vi "Main.vi"() -> ()   [LabVIEW 2013]
uses:
  <vilib>/Utility/error.llb/DialogType.ctl
panel:
  in  "Boolean":bool
  in  "Set Output ON All":bool
  in  "Set Output OFF All":bool
  out "CURRENTSET":dbl[](array[numeric])
  in  "CurrentModulationOn":bool
  in  "Amp":dbl
  in  "CurrentModulationB":bool
  in  "ModulationUpDown":bool
  in  "ModulationNumberOfSteps":i32
  in  "ModulationState":i32
  in  "Step":dbl
  in  "Period":u32
  in  "ConnectAll":bool
  in  "DisconnectAll":bool
  in  "SetCurrentAll":bool
  in  "SetVoltageAll":bool
  in  "SetOutputOffB":bool
  in  "SetOutputOnB":bool
  in  "ReadFromFile":bool
  in  "Name":string="55"
  out "NAME":string[](array[string])
  in  "WriteToFile":bool
  in  "SetCurrent":dbl step=0.1
  in  "SetVoltage":dbl
  in  "SetCurrentB":bool
  in  "SetVoltageB":bool
  in  "DeleteChannel":bool
  in  "ConnectChannel":bool
  in  "DisconnectChannel":bool
  out "ADRESS":string[](array[string])
  out "VIRef":refnum<vi>[](array[refnum])
  in  "Quit":bool
  in  "List of channels":i32(listbox)
  in  "IP":string="172.16.21.19"
  in  "AddChannel":bool
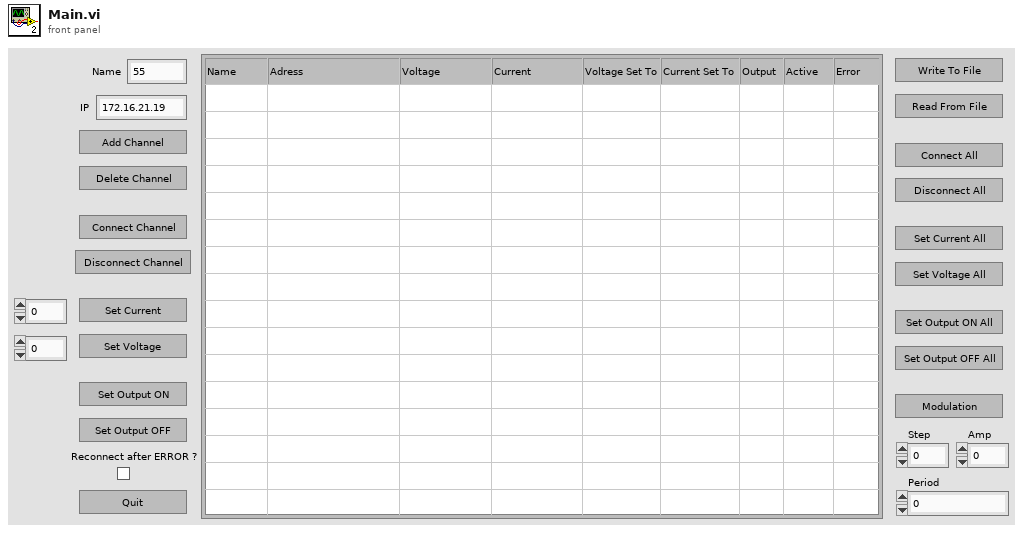
[diagram p1: front panel]
types:
  T1 = typedef "DialogType.ctl" = u16
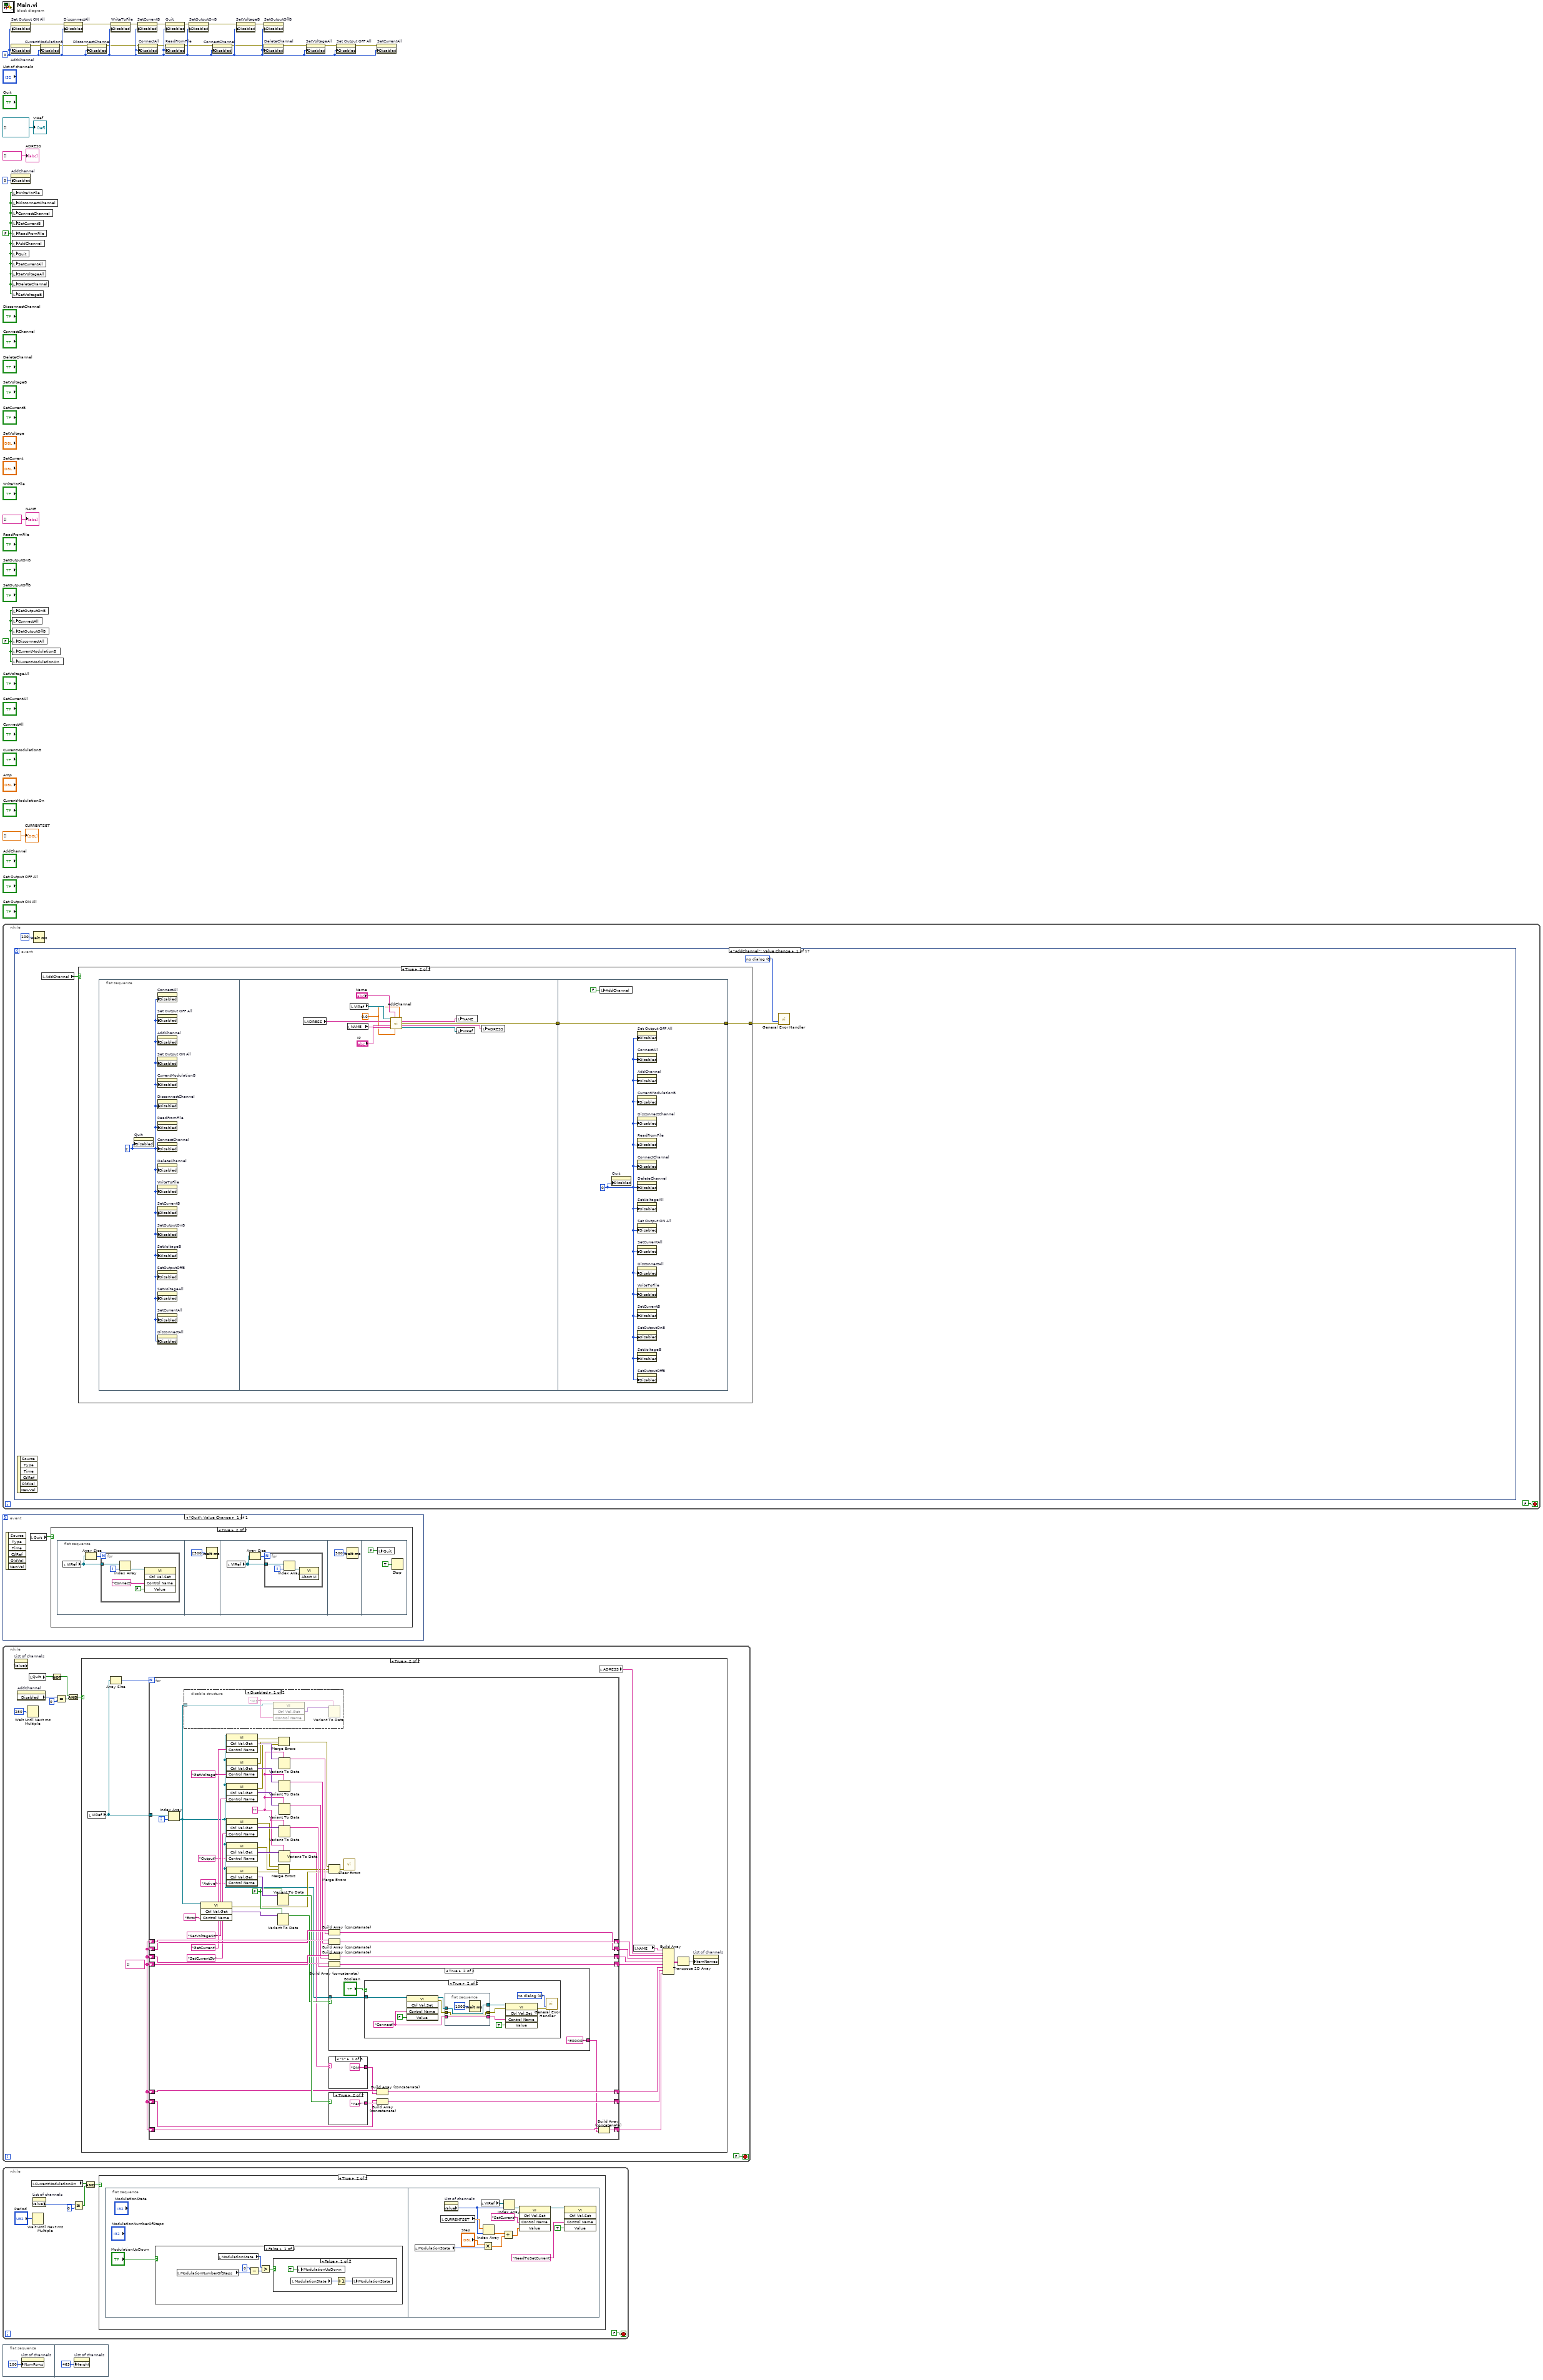
[diagram p0: block diagram]
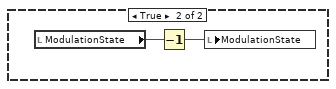
[diagram p3: hidden frame]
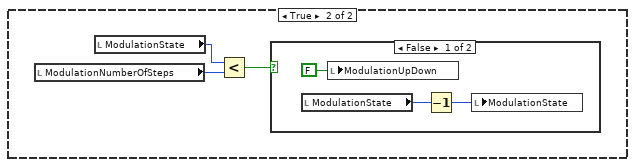
[diagram p4: hidden frame]
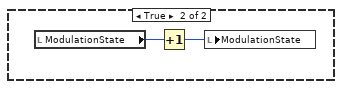
[diagram p5: hidden frame]
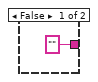
[diagram p8: hidden frame]
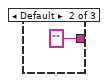
[diagram p10: hidden frame]
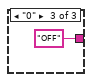
[diagram p11: hidden frame]
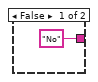
[diagram p12: hidden frame]
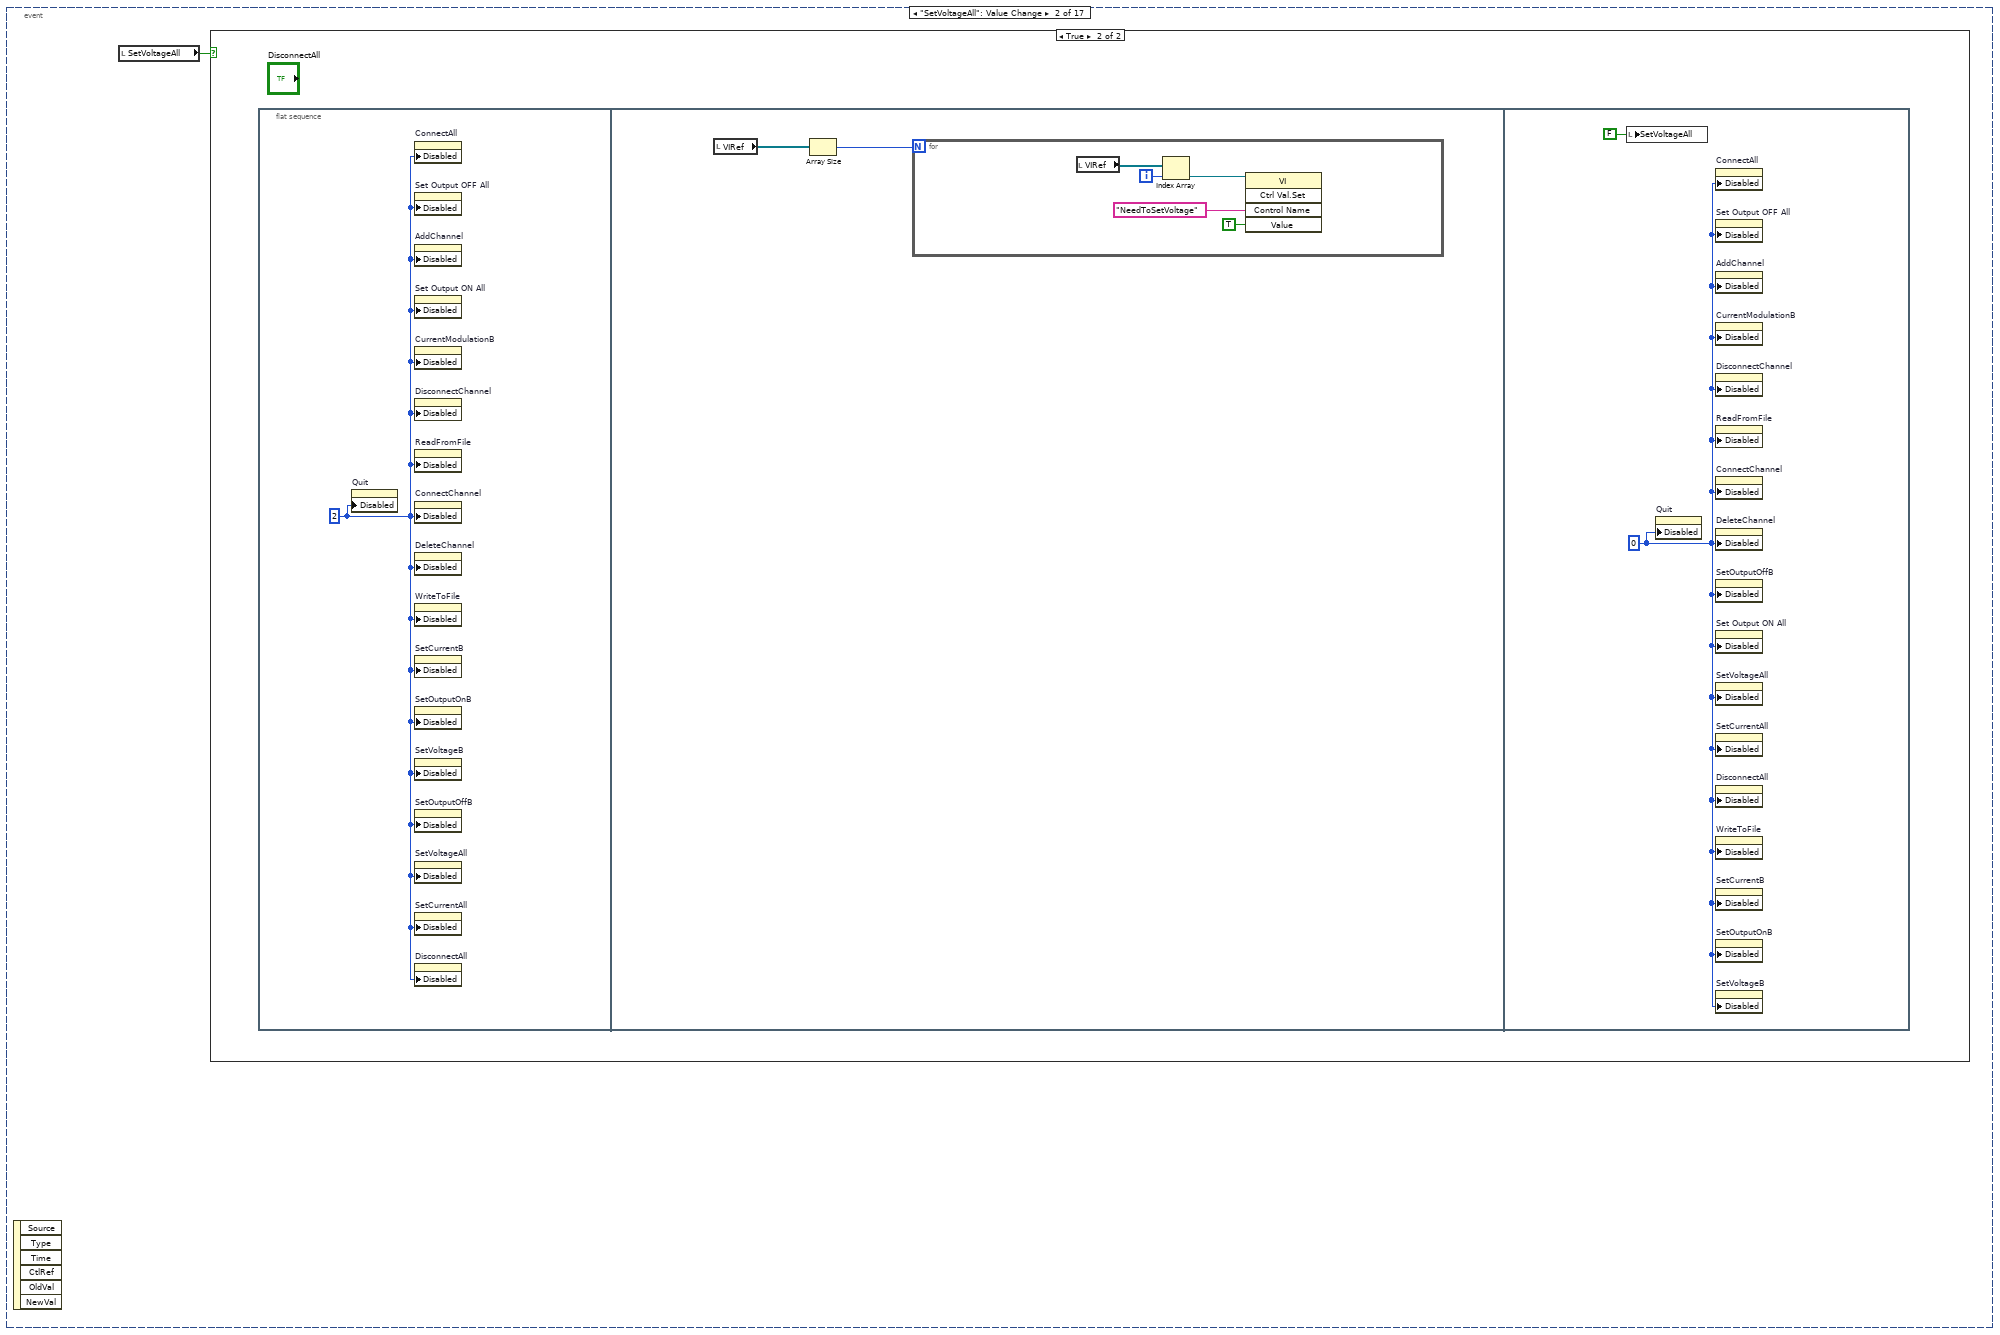
[diagram p15: hidden frame]
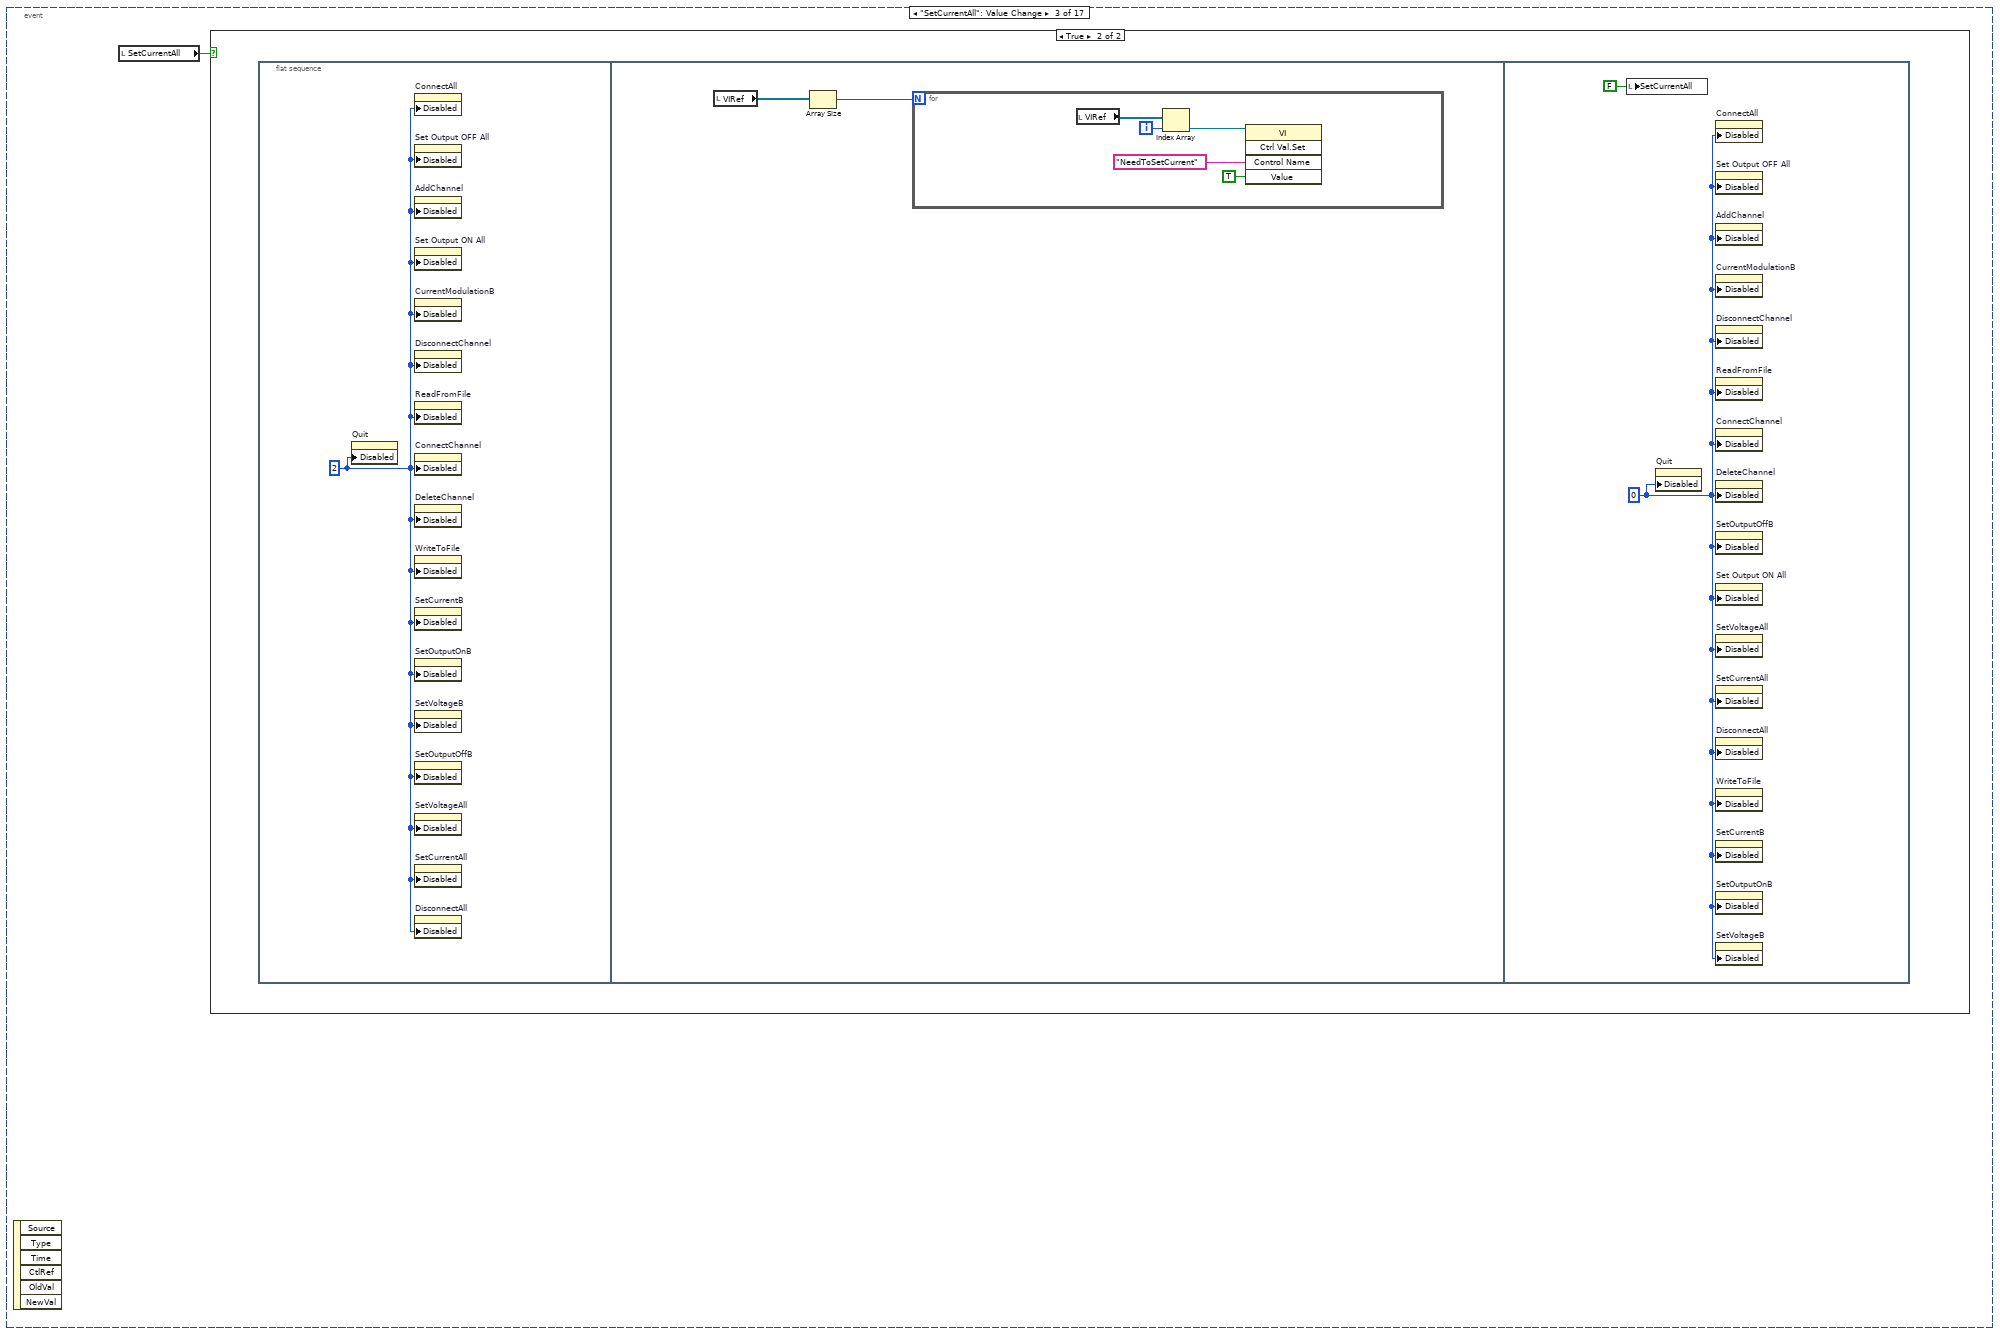
[diagram p17: hidden frame]
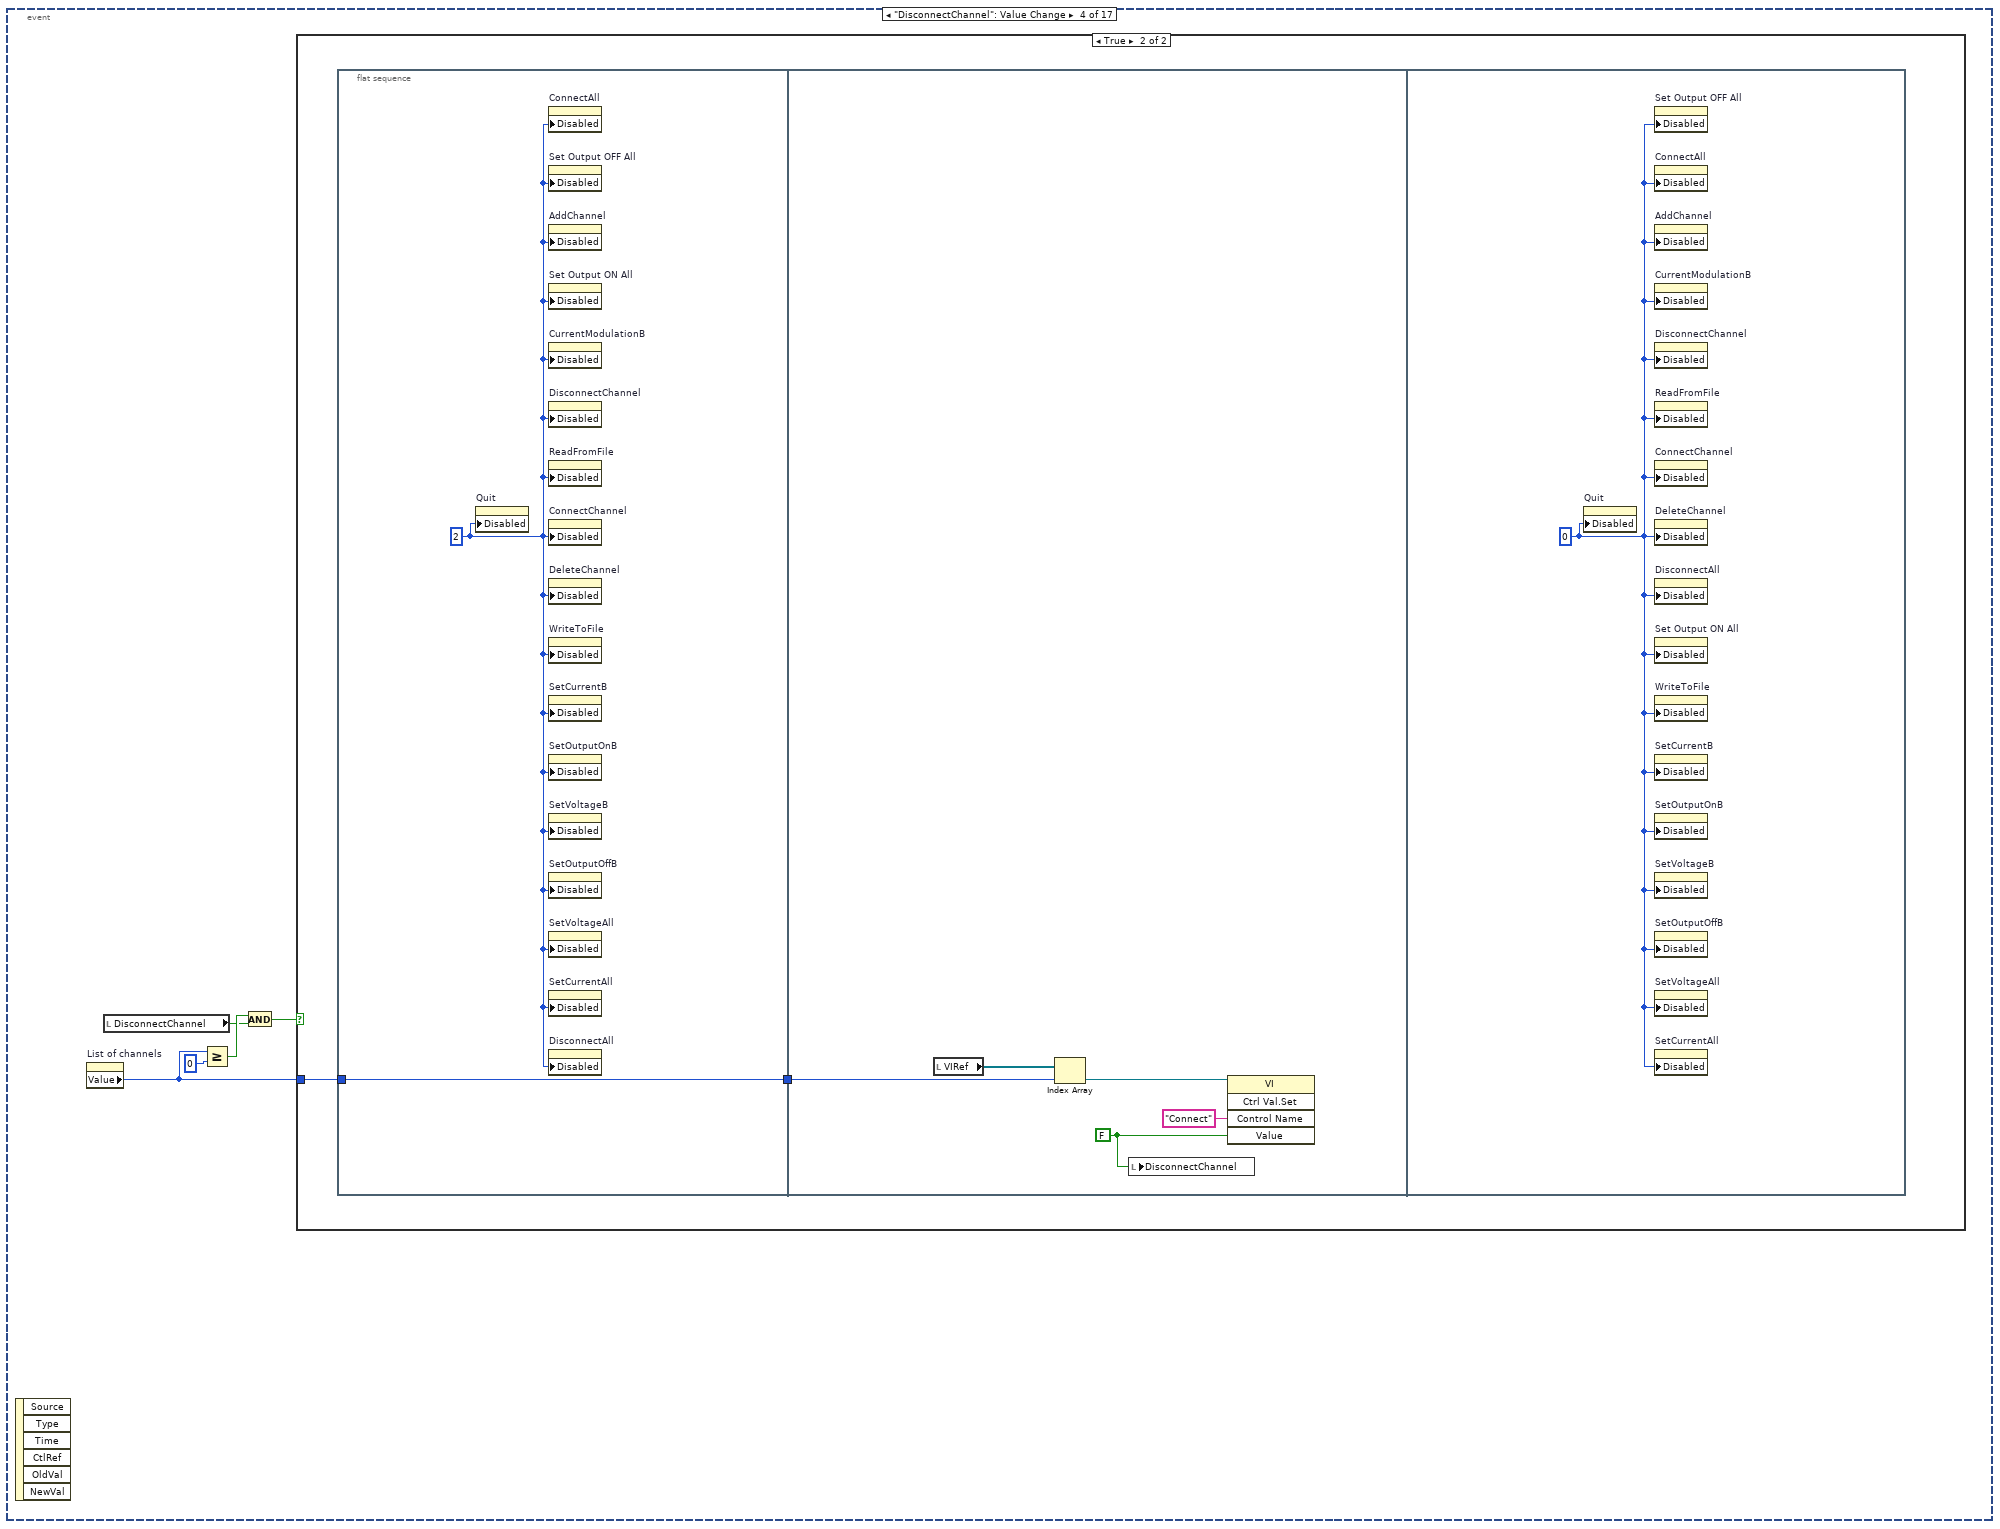
[diagram p19: hidden frame]
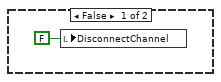
[diagram p20: hidden frame]
diagram:
  w17 = u8 0 ("Disabled")
  w19 = FALSE ("SetOutputOnB")
  w20 = FALSE ("OK Button")
  n1 = while {
    stop <- FALSE stop-if-true
    n2 = event shown="[0] \"AddChannel\": Value Change" {
      selector: _ -> [_ _ _ _ _ _ _ _ _ _ _ _ _ _ _ _ _]
      dyn-events: _ -> [_ _ _ _ _ _ _ _ _ _ _ _ _ _ _ _ _]
      timeout: _ -> [_ _ _ _ _ _ _ _ _ _ _ _ _ _ _ _ _]
      event "AddChannel": Value Change {
        w27 = T1 0 items=["no dialog", "OK message", "continue or stop message", "OK message + warnings", "continue/stop + warnings"] ("type of dialog (OK msg:1)")
        n3 = event-data() -> ()  [unwired: 7 out]
        n4 = local read "AddChannel"() -> (w29:bool)
        n5 = case shown="True" w29 {
          tunnel: [_ w30] -> w28
          frame False {
          }
          frame True {
            n6 = flat-sequence {
              tunnel: [w33] -> w31
              tunnel: [w43] -> w30
              tunnel: w31 -> [w43]
              frame #0 {
                w32 = u8 2 ("Disabled")
                n7 = property on="Quit" class="Bool (strict)"("Disabled"=w32) -> ()  [unwired: 2 in, 2 out]
                n8 = property on="ConnectAll" class="Bool (strict)"("Disabled"=w32) -> ()  [unwired: 2 in, 2 out]
                n9 = property on="Set Output OFF All" class="Bool (strict)"("Disabled"=w32) -> ()  [unwired: 2 in, 2 out]
                n10 = property on="AddChannel" class="Bool (strict)"("Disabled"=w32) -> ()  [unwired: 2 in, 2 out]
                n11 = property on="Set Output ON All" class="Bool (strict)"("Disabled"=w32) -> ()  [unwired: 2 in, 2 out]
                n12 = property on="CurrentModulationB" class="Bool (strict)"("Disabled"=w32) -> ()  [unwired: 2 in, 2 out]
                n13 = property on="DisconnectChannel" class="Bool (strict)"("Disabled"=w32) -> ()  [unwired: 2 in, 2 out]
                n14 = property on="ReadFromFile" class="Bool (strict)"("Disabled"=w32) -> ()  [unwired: 2 in, 2 out]
                n15 = property on="ConnectChannel" class="Bool (strict)"("Disabled"=w32) -> ()  [unwired: 2 in, 2 out]
                n16 = property on="DeleteChannel" class="Bool (strict)"("Disabled"=w32) -> ()  [unwired: 2 in, 2 out]
                n17 = property on="WriteToFile" class="Bool (strict)"("Disabled"=w32) -> ()  [unwired: 2 in, 2 out]
                n18 = property on="SetCurrentB" class="Bool (strict)"("Disabled"=w32) -> ()  [unwired: 2 in, 2 out]
                n19 = property on="SetOutputOnB" class="Bool (strict)"("Disabled"=w32) -> ()  [unwired: 2 in, 2 out]
                n20 = property on="SetVoltageB" class="Bool (strict)"("Disabled"=w32) -> ()  [unwired: 2 in, 2 out]
                n21 = property on="SetOutputOffB" class="Bool (strict)"("Disabled"=w32) -> ()  [unwired: 2 in, 2 out]
                n22 = property on="SetVoltageAll" class="Bool (strict)"("Disabled"=w32) -> ()  [unwired: 2 in, 2 out]
                n23 = property on="SetCurrentAll" class="Bool (strict)"("Disabled"=w32) -> ()  [unwired: 2 in, 2 out]
                n24 = property on="DisconnectAll" class="Bool (strict)"("Disabled"=w32) -> ()  [unwired: 2 in, 2 out]
              }
              frame #1 {
                w34 = 0.0 ("SetVoltage")
                n25 = local read "ADRESS"() -> (w40:string[])
                n26 = local read "NAME"() -> (w39:string[])
                n27 = local read "VIRef"() -> (w38:refnum<vi>[])
                n28 = call "AddChannel.vi"("VIRef"=w38, "Name"="Name", "SetCurrent"=w34, "ADRESS"=w40, "NAME"=w39, "Address"="IP", "SetVoltage"=w34) -> ("NAMEOut"=w35:string[], "error out"=w33:errorcluster, "ADRESSOut"=w36:string[], "VIRefOut"=w37:refnum<vi>[])  [unwired: 1 in, 4 out]
                n29 = local write "NAME"(w35) -> ()
                n30 = local write "VIRef"(w37) -> ()
                n31 = local write "ADRESS"(w36) -> ()
              }
              frame #2 {
                w44 = u8 0 ("Disabled")
                n32 = local write "AddChannel"(FALSE ("AddChannel")) -> ()
                n33 = property on="Quit" class="Bool (strict)"("Disabled"=w44) -> ()  [unwired: 2 in, 2 out]
                n34 = property on="Set Output OFF All" class="Bool (strict)"("Disabled"=w44) -> ()  [unwired: 2 in, 2 out]
                n35 = property on="ConnectAll" class="Bool (strict)"("Disabled"=w44) -> ()  [unwired: 2 in, 2 out]
                n36 = property on="AddChannel" class="Bool (strict)"("Disabled"=w44) -> ()  [unwired: 2 in, 2 out]
                n37 = property on="CurrentModulationB" class="Bool (strict)"("Disabled"=w44) -> ()  [unwired: 2 in, 2 out]
                n38 = property on="DisconnectChannel" class="Bool (strict)"("Disabled"=w44) -> ()  [unwired: 2 in, 2 out]
                n39 = property on="ReadFromFile" class="Bool (strict)"("Disabled"=w44) -> ()  [unwired: 2 in, 2 out]
                n40 = property on="ConnectChannel" class="Bool (strict)"("Disabled"=w44) -> ()  [unwired: 2 in, 2 out]
                n41 = property on="DeleteChannel" class="Bool (strict)"("Disabled"=w44) -> ()  [unwired: 2 in, 2 out]
                n42 = property on="SetVoltageAll" class="Bool (strict)"("Disabled"=w44) -> ()  [unwired: 2 in, 2 out]
                n43 = property on="Set Output ON All" class="Bool (strict)"("Disabled"=w44) -> ()  [unwired: 2 in, 2 out]
                n44 = property on="SetCurrentAll" class="Bool (strict)"("Disabled"=w44) -> ()  [unwired: 2 in, 2 out]
                n45 = property on="DisconnectAll" class="Bool (strict)"("Disabled"=w44) -> ()  [unwired: 2 in, 2 out]
                n46 = property on="WriteToFile" class="Bool (strict)"("Disabled"=w44) -> ()  [unwired: 2 in, 2 out]
                n47 = property on="SetCurrentB" class="Bool (strict)"("Disabled"=w44) -> ()  [unwired: 2 in, 2 out]
                n48 = property on="SetOutputOnB" class="Bool (strict)"("Disabled"=w44) -> ()  [unwired: 2 in, 2 out]
                n49 = property on="SetVoltageB" class="Bool (strict)"("Disabled"=w44) -> ()  [unwired: 2 in, 2 out]
                n50 = property on="SetOutputOffB" class="Bool (strict)"("Disabled"=w44) -> ()  [unwired: 2 in, 2 out]
              }
            }
          }
        }
        n51 = call <vilib>:"General Error Handler.vi"("type of dialog (OK msg:1)"=w27, "error in (no error)"=w28) -> ()  [unwired: 14 out]
      }
      event "SetVoltageAll": Value Change {
        n52 = event-data() -> ()  [unwired: 7 out]
        n53 = local read "SetVoltageAll"() -> (w46:bool)
        n54 = case shown="True" w46 {
          frame False {
          }
          frame True {
            n55 = flat-sequence {
              frame #0 {
                w47 = u8 2 ("Disabled")
                n56 = property on="Quit" class="Bool (strict)"("Disabled"=w47) -> ()  [unwired: 2 in, 2 out]
                n57 = property on="ConnectAll" class="Bool (strict)"("Disabled"=w47) -> ()  [unwired: 2 in, 2 out]
                n58 = property on="Set Output OFF All" class="Bool (strict)"("Disabled"=w47) -> ()  [unwired: 2 in, 2 out]
                n59 = property on="AddChannel" class="Bool (strict)"("Disabled"=w47) -> ()  [unwired: 2 in, 2 out]
                n60 = property on="Set Output ON All" class="Bool (strict)"("Disabled"=w47) -> ()  [unwired: 2 in, 2 out]
                n61 = property on="CurrentModulationB" class="Bool (strict)"("Disabled"=w47) -> ()  [unwired: 2 in, 2 out]
                n62 = property on="DisconnectChannel" class="Bool (strict)"("Disabled"=w47) -> ()  [unwired: 2 in, 2 out]
                n63 = property on="ReadFromFile" class="Bool (strict)"("Disabled"=w47) -> ()  [unwired: 2 in, 2 out]
                n64 = property on="ConnectChannel" class="Bool (strict)"("Disabled"=w47) -> ()  [unwired: 2 in, 2 out]
                n65 = property on="DeleteChannel" class="Bool (strict)"("Disabled"=w47) -> ()  [unwired: 2 in, 2 out]
                n66 = property on="WriteToFile" class="Bool (strict)"("Disabled"=w47) -> ()  [unwired: 2 in, 2 out]
                n67 = property on="SetCurrentB" class="Bool (strict)"("Disabled"=w47) -> ()  [unwired: 2 in, 2 out]
                n68 = property on="SetOutputOnB" class="Bool (strict)"("Disabled"=w47) -> ()  [unwired: 2 in, 2 out]
                n69 = property on="SetVoltageB" class="Bool (strict)"("Disabled"=w47) -> ()  [unwired: 2 in, 2 out]
                n70 = property on="SetOutputOffB" class="Bool (strict)"("Disabled"=w47) -> ()  [unwired: 2 in, 2 out]
                n71 = property on="SetVoltageAll" class="Bool (strict)"("Disabled"=w47) -> ()  [unwired: 2 in, 2 out]
                n72 = property on="SetCurrentAll" class="Bool (strict)"("Disabled"=w47) -> ()  [unwired: 2 in, 2 out]
                n73 = property on="DisconnectAll" class="Bool (strict)"("Disabled"=w47) -> ()  [unwired: 2 in, 2 out]
              }
              frame #1 {
                n74 = local read "VIRef"() -> (w49:refnum<vi>[])
                n75 = Array Size(array=w49) -> (size(s)=w48:i32)
                n76 = for {
                  N: w48 -> [_]
                  i -> [w51]
                  n77 = local read "VIRef"() -> (w54:refnum<vi>[])
                  n78 = Index Array(array=w54, index=w51) -> (element=w50:refnum<vi>)
                  n79 = invoke class="VI" method="Ctrl Val.Set"(reference=w50, "Control Name"="NeedToSetVoltage", "Value"=TRUE ("ConnectChannel")) -> ()  [unwired: 2 in, 5 out]
                }
              }
              frame #2 {
                w55 = u8 0 ("Disabled")
                n80 = local write "SetVoltageAll"(FALSE ("SetVoltageAll")) -> ()
                n81 = property on="Quit" class="Bool (strict)"("Disabled"=w55) -> ()  [unwired: 2 in, 2 out]
                n82 = property on="ConnectAll" class="Bool (strict)"("Disabled"=w55) -> ()  [unwired: 2 in, 2 out]
                n83 = property on="Set Output OFF All" class="Bool (strict)"("Disabled"=w55) -> ()  [unwired: 2 in, 2 out]
                n84 = property on="AddChannel" class="Bool (strict)"("Disabled"=w55) -> ()  [unwired: 2 in, 2 out]
                n85 = property on="CurrentModulationB" class="Bool (strict)"("Disabled"=w55) -> ()  [unwired: 2 in, 2 out]
                n86 = property on="DisconnectChannel" class="Bool (strict)"("Disabled"=w55) -> ()  [unwired: 2 in, 2 out]
                n87 = property on="ReadFromFile" class="Bool (strict)"("Disabled"=w55) -> ()  [unwired: 2 in, 2 out]
                n88 = property on="ConnectChannel" class="Bool (strict)"("Disabled"=w55) -> ()  [unwired: 2 in, 2 out]
                n89 = property on="DeleteChannel" class="Bool (strict)"("Disabled"=w55) -> ()  [unwired: 2 in, 2 out]
                n90 = property on="SetOutputOffB" class="Bool (strict)"("Disabled"=w55) -> ()  [unwired: 2 in, 2 out]
                n91 = property on="Set Output ON All" class="Bool (strict)"("Disabled"=w55) -> ()  [unwired: 2 in, 2 out]
                n92 = property on="SetVoltageAll" class="Bool (strict)"("Disabled"=w55) -> ()  [unwired: 2 in, 2 out]
                n93 = property on="SetCurrentAll" class="Bool (strict)"("Disabled"=w55) -> ()  [unwired: 2 in, 2 out]
                n94 = property on="DisconnectAll" class="Bool (strict)"("Disabled"=w55) -> ()  [unwired: 2 in, 2 out]
                n95 = property on="WriteToFile" class="Bool (strict)"("Disabled"=w55) -> ()  [unwired: 2 in, 2 out]
                n96 = property on="SetCurrentB" class="Bool (strict)"("Disabled"=w55) -> ()  [unwired: 2 in, 2 out]
                n97 = property on="SetOutputOnB" class="Bool (strict)"("Disabled"=w55) -> ()  [unwired: 2 in, 2 out]
                n98 = property on="SetVoltageB" class="Bool (strict)"("Disabled"=w55) -> ()  [unwired: 2 in, 2 out]
              }
            }
          }
        }
      }
      event "SetCurrentAll": Value Change {
        n99 = event-data() -> ()  [unwired: 7 out]
        n100 = local read "SetCurrentAll"() -> (w57:bool)
        n101 = case shown="True" w57 {
          frame False {
          }
          frame True {
            n102 = flat-sequence {
              frame #0 {
                w58 = u8 2 ("Disabled")
                n103 = property on="Quit" class="Bool (strict)"("Disabled"=w58) -> ()  [unwired: 2 in, 2 out]
                n104 = property on="ConnectAll" class="Bool (strict)"("Disabled"=w58) -> ()  [unwired: 2 in, 2 out]
                n105 = property on="Set Output OFF All" class="Bool (strict)"("Disabled"=w58) -> ()  [unwired: 2 in, 2 out]
                n106 = property on="AddChannel" class="Bool (strict)"("Disabled"=w58) -> ()  [unwired: 2 in, 2 out]
                n107 = property on="Set Output ON All" class="Bool (strict)"("Disabled"=w58) -> ()  [unwired: 2 in, 2 out]
                n108 = property on="CurrentModulationB" class="Bool (strict)"("Disabled"=w58) -> ()  [unwired: 2 in, 2 out]
                n109 = property on="DisconnectChannel" class="Bool (strict)"("Disabled"=w58) -> ()  [unwired: 2 in, 2 out]
                n110 = property on="ReadFromFile" class="Bool (strict)"("Disabled"=w58) -> ()  [unwired: 2 in, 2 out]
                n111 = property on="ConnectChannel" class="Bool (strict)"("Disabled"=w58) -> ()  [unwired: 2 in, 2 out]
                n112 = property on="DeleteChannel" class="Bool (strict)"("Disabled"=w58) -> ()  [unwired: 2 in, 2 out]
                n113 = property on="WriteToFile" class="Bool (strict)"("Disabled"=w58) -> ()  [unwired: 2 in, 2 out]
                n114 = property on="SetCurrentB" class="Bool (strict)"("Disabled"=w58) -> ()  [unwired: 2 in, 2 out]
                n115 = property on="SetOutputOnB" class="Bool (strict)"("Disabled"=w58) -> ()  [unwired: 2 in, 2 out]
                n116 = property on="SetVoltageB" class="Bool (strict)"("Disabled"=w58) -> ()  [unwired: 2 in, 2 out]
                n117 = property on="SetOutputOffB" class="Bool (strict)"("Disabled"=w58) -> ()  [unwired: 2 in, 2 out]
                n118 = property on="SetVoltageAll" class="Bool (strict)"("Disabled"=w58) -> ()  [unwired: 2 in, 2 out]
                n119 = property on="SetCurrentAll" class="Bool (strict)"("Disabled"=w58) -> ()  [unwired: 2 in, 2 out]
                n120 = property on="DisconnectAll" class="Bool (strict)"("Disabled"=w58) -> ()  [unwired: 2 in, 2 out]
              }
              frame #1 {
                n121 = local read "VIRef"() -> (w60:refnum<vi>[])
                n122 = Array Size(array=w60) -> (size(s)=w59:i32)
                n123 = for {
                  N: w59 -> [_]
                  i -> [w62]
                  n124 = local read "VIRef"() -> (w65:refnum<vi>[])
                  n125 = Index Array(array=w65, index=w62) -> (element=w61:refnum<vi>)
                  n126 = invoke class="VI" method="Ctrl Val.Set"(reference=w61, "Control Name"="NeedToSetCurrent", "Value"=TRUE ("ConnectChannel")) -> ()  [unwired: 2 in, 5 out]
                }
              }
              frame #2 {
                w66 = u8 0 ("Disabled")
                n127 = local write "SetCurrentAll"(FALSE ("SetVoltageAll")) -> ()
                n128 = property on="Quit" class="Bool (strict)"("Disabled"=w66) -> ()  [unwired: 2 in, 2 out]
                n129 = property on="ConnectAll" class="Bool (strict)"("Disabled"=w66) -> ()  [unwired: 2 in, 2 out]
                n130 = property on="Set Output OFF All" class="Bool (strict)"("Disabled"=w66) -> ()  [unwired: 2 in, 2 out]
                n131 = property on="AddChannel" class="Bool (strict)"("Disabled"=w66) -> ()  [unwired: 2 in, 2 out]
                n132 = property on="CurrentModulationB" class="Bool (strict)"("Disabled"=w66) -> ()  [unwired: 2 in, 2 out]
                n133 = property on="DisconnectChannel" class="Bool (strict)"("Disabled"=w66) -> ()  [unwired: 2 in, 2 out]
                n134 = property on="ReadFromFile" class="Bool (strict)"("Disabled"=w66) -> ()  [unwired: 2 in, 2 out]
                n135 = property on="ConnectChannel" class="Bool (strict)"("Disabled"=w66) -> ()  [unwired: 2 in, 2 out]
                n136 = property on="DeleteChannel" class="Bool (strict)"("Disabled"=w66) -> ()  [unwired: 2 in, 2 out]
                n137 = property on="SetOutputOffB" class="Bool (strict)"("Disabled"=w66) -> ()  [unwired: 2 in, 2 out]
                n138 = property on="Set Output ON All" class="Bool (strict)"("Disabled"=w66) -> ()  [unwired: 2 in, 2 out]
                n139 = property on="SetVoltageAll" class="Bool (strict)"("Disabled"=w66) -> ()  [unwired: 2 in, 2 out]
                n140 = property on="SetCurrentAll" class="Bool (strict)"("Disabled"=w66) -> ()  [unwired: 2 in, 2 out]
                n141 = property on="DisconnectAll" class="Bool (strict)"("Disabled"=w66) -> ()  [unwired: 2 in, 2 out]
                n142 = property on="WriteToFile" class="Bool (strict)"("Disabled"=w66) -> ()  [unwired: 2 in, 2 out]
                n143 = property on="SetCurrentB" class="Bool (strict)"("Disabled"=w66) -> ()  [unwired: 2 in, 2 out]
                n144 = property on="SetOutputOnB" class="Bool (strict)"("Disabled"=w66) -> ()  [unwired: 2 in, 2 out]
                n145 = property on="SetVoltageB" class="Bool (strict)"("Disabled"=w66) -> ()  [unwired: 2 in, 2 out]
              }
            }
          }
        }
      }
      event "DisconnectChannel": Value Change {
        n146 = event-data() -> ()  [unwired: 7 out]
        n147 = property on="List of channels" class="MCListbox (strict)"() -> ("Value"=w68:i32)  [unwired: 2 in, 2 out]
        n148 = local read "DisconnectChannel"() -> (w69:bool)
        n149 = Greater Or Equal?(x=w68, y=0) -> (x >= y?=w72:bool)
        n150 = And(x=w72, y=w69) -> (x .and. y?=w70:bool)
        n151 = case shown="True" w70 {
          tunnel: w68 -> [_ w75]
          frame False {
            n152 = local write "DisconnectChannel"(FALSE ("DisconnectChannel")) -> ()
          }
          frame True {
            n153 = flat-sequence {
              tunnel: w75 -> [w77]
              tunnel: [w77] -> w74
              tunnel: w74 -> [w78]
              frame #0 {
                w76 = u8 2 ("Disabled")
                n154 = property on="Quit" class="Bool (strict)"("Disabled"=w76) -> ()  [unwired: 2 in, 2 out]
                n155 = property on="ConnectAll" class="Bool (strict)"("Disabled"=w76) -> ()  [unwired: 2 in, 2 out]
                n156 = property on="Set Output OFF All" class="Bool (strict)"("Disabled"=w76) -> ()  [unwired: 2 in, 2 out]
                n157 = property on="AddChannel" class="Bool (strict)"("Disabled"=w76) -> ()  [unwired: 2 in, 2 out]
                n158 = property on="Set Output ON All" class="Bool (strict)"("Disabled"=w76) -> ()  [unwired: 2 in, 2 out]
                n159 = property on="CurrentModulationB" class="Bool (strict)"("Disabled"=w76) -> ()  [unwired: 2 in, 2 out]
                n160 = property on="DisconnectChannel" class="Bool (strict)"("Disabled"=w76) -> ()  [unwired: 2 in, 2 out]
                n161 = property on="ReadFromFile" class="Bool (strict)"("Disabled"=w76) -> ()  [unwired: 2 in, 2 out]
                n162 = property on="ConnectChannel" class="Bool (strict)"("Disabled"=w76) -> ()  [unwired: 2 in, 2 out]
                n163 = property on="DeleteChannel" class="Bool (strict)"("Disabled"=w76) -> ()  [unwired: 2 in, 2 out]
                n164 = property on="WriteToFile" class="Bool (strict)"("Disabled"=w76) -> ()  [unwired: 2 in, 2 out]
                n165 = property on="SetCurrentB" class="Bool (strict)"("Disabled"=w76) -> ()  [unwired: 2 in, 2 out]
                n166 = property on="SetOutputOnB" class="Bool (strict)"("Disabled"=w76) -> ()  [unwired: 2 in, 2 out]
                n167 = property on="SetVoltageB" class="Bool (strict)"("Disabled"=w76) -> ()  [unwired: 2 in, 2 out]
                n168 = property on="SetOutputOffB" class="Bool (strict)"("Disabled"=w76) -> ()  [unwired: 2 in, 2 out]
                n169 = property on="SetVoltageAll" class="Bool (strict)"("Disabled"=w76) -> ()  [unwired: 2 in, 2 out]
                n170 = property on="SetCurrentAll" class="Bool (strict)"("Disabled"=w76) -> ()  [unwired: 2 in, 2 out]
                n171 = property on="DisconnectAll" class="Bool (strict)"("Disabled"=w76) -> ()  [unwired: 2 in, 2 out]
              }
              frame #1 {
                w79 = FALSE ("OK Button")
                n172 = local read "VIRef"() -> (w81:refnum<vi>[])
                n173 = Index Array(array=w81, index=w78) -> (element=w80:refnum<vi>)
                n174 = local write "DisconnectChannel"(w79) -> ()
                n175 = invoke class="VI" method="Ctrl Val.Set"(reference=w80, "Control Name"="Connect", "Value"=w79) -> ()  [unwired: 2 in, 5 out]
              }
              frame #2 {
                w83 = u8 0 ("Disabled")
                n176 = property on="Quit" class="Bool (strict)"("Disabled"=w83) -> ()  [unwired: 2 in, 2 out]
                n177 = property on="Set Output OFF All" class="Bool (strict)"("Disabled"=w83) -> ()  [unwired: 2 in, 2 out]
                n178 = property on="ConnectAll" class="Bool (strict)"("Disabled"=w83) -> ()  [unwired: 2 in, 2 out]
                n179 = property on="AddChannel" class="Bool (strict)"("Disabled"=w83) -> ()  [unwired: 2 in, 2 out]
                n180 = property on="CurrentModulationB" class="Bool (strict)"("Disabled"=w83) -> ()  [unwired: 2 in, 2 out]
                n181 = property on="DisconnectChannel" class="Bool (strict)"("Disabled"=w83) -> ()  [unwired: 2 in, 2 out]
                n182 = property on="ReadFromFile" class="Bool (strict)"("Disabled"=w83) -> ()  [unwired: 2 in, 2 out]
                n183 = property on="ConnectChannel" class="Bool (strict)"("Disabled"=w83) -> ()  [unwired: 2 in, 2 out]
                n184 = property on="DeleteChannel" class="Bool (strict)"("Disabled"=w83) -> ()  [unwired: 2 in, 2 out]
                n185 = property on="DisconnectAll" class="Bool (strict)"("Disabled"=w83) -> ()  [unwired: 2 in, 2 out]
                n186 = property on="Set Output ON All" class="Bool (strict)"("Disabled"=w83) -> ()  [unwired: 2 in, 2 out]
                n187 = property on="WriteToFile" class="Bool (strict)"("Disabled"=w83) -> ()  [unwired: 2 in, 2 out]
                n188 = property on="SetCurrentB" class="Bool (strict)"("Disabled"=w83) -> ()  [unwired: 2 in, 2 out]
                n189 = property on="SetOutputOnB" class="Bool (strict)"("Disabled"=w83) -> ()  [unwired: 2 in, 2 out]
                n190 = property on="SetVoltageB" class="Bool (strict)"("Disabled"=w83) -> ()  [unwired: 2 in, 2 out]
                n191 = property on="SetOutputOffB" class="Bool (strict)"("Disabled"=w83) -> ()  [unwired: 2 in, 2 out]
                n192 = property on="SetVoltageAll" class="Bool (strict)"("Disabled"=w83) -> ()  [unwired: 2 in, 2 out]
                n193 = property on="SetCurrentAll" class="Bool (strict)"("Disabled"=w83) -> ()  [unwired: 2 in, 2 out]
              }
            }
          }
        }
      }
      event "ConnectChannel": Value Change {
        n194 = event-data() -> ()  [unwired: 7 out]
        n195 = property on="List of channels" class="MCListbox (strict)"() -> ("Value"=w84:i32)  [unwired: 2 in, 2 out]
        n196 = local read "ConnectChannel"() -> (w85:bool)
        n197 = Greater Or Equal?(x=w84, y=0) -> (x >= y?=w87:bool)
        n198 = And(x=w87, y=w85) -> (x .and. y?=w86:bool)
        n199 = case shown="True" w86 {
          tunnel: w84 -> [_ w91]
          frame False {
            n200 = local write "ConnectChannel"(FALSE ("ConnectChannel")) -> ()
          }
          frame True {
            n201 = flat-sequence {
              tunnel: w91 -> [w93]
              tunnel: [w93] -> w90
              tunnel: w90 -> [w94]
              frame #0 {
                w92 = u8 2 ("Disabled")
                n202 = property on="Quit" class="Bool (strict)"("Disabled"=w92) -> ()  [unwired: 2 in, 2 out]
                n203 = property on="ConnectAll" class="Bool (strict)"("Disabled"=w92) -> ()  [unwired: 2 in, 2 out]
                n204 = property on="Set Output OFF All" class="Bool (strict)"("Disabled"=w92) -> ()  [unwired: 2 in, 2 out]
                n205 = property on="AddChannel" class="Bool (strict)"("Disabled"=w92) -> ()  [unwired: 2 in, 2 out]
                n206 = property on="Set Output ON All" class="Bool (strict)"("Disabled"=w92) -> ()  [unwired: 2 in, 2 out]
                n207 = property on="CurrentModulationB" class="Bool (strict)"("Disabled"=w92) -> ()  [unwired: 2 in, 2 out]
                n208 = property on="DisconnectChannel" class="Bool (strict)"("Disabled"=w92) -> ()  [unwired: 2 in, 2 out]
                n209 = property on="ReadFromFile" class="Bool (strict)"("Disabled"=w92) -> ()  [unwired: 2 in, 2 out]
                n210 = property on="ConnectChannel" class="Bool (strict)"("Disabled"=w92) -> ()  [unwired: 2 in, 2 out]
                n211 = property on="DeleteChannel" class="Bool (strict)"("Disabled"=w92) -> ()  [unwired: 2 in, 2 out]
                n212 = property on="WriteToFile" class="Bool (strict)"("Disabled"=w92) -> ()  [unwired: 2 in, 2 out]
                n213 = property on="SetCurrentB" class="Bool (strict)"("Disabled"=w92) -> ()  [unwired: 2 in, 2 out]
                n214 = property on="SetOutputOnB" class="Bool (strict)"("Disabled"=w92) -> ()  [unwired: 2 in, 2 out]
                n215 = property on="SetVoltageB" class="Bool (strict)"("Disabled"=w92) -> ()  [unwired: 2 in, 2 out]
                n216 = property on="SetOutputOffB" class="Bool (strict)"("Disabled"=w92) -> ()  [unwired: 2 in, 2 out]
                n217 = property on="SetVoltageAll" class="Bool (strict)"("Disabled"=w92) -> ()  [unwired: 2 in, 2 out]
                n218 = property on="SetCurrentAll" class="Bool (strict)"("Disabled"=w92) -> ()  [unwired: 2 in, 2 out]
                n219 = property on="DisconnectAll" class="Bool (strict)"("Disabled"=w92) -> ()  [unwired: 2 in, 2 out]
              }
              frame #1 {
                n220 = local read "VIRef"() -> (w97:refnum<vi>[])
                n221 = Index Array(array=w97, index=w94) -> (element=w96:refnum<vi>)
                n222 = invoke class="VI" method="Ctrl Val.Set"(reference=w96, "Control Name"="Connect", "Value"=TRUE ("OK Button")) -> ()  [unwired: 2 in, 5 out]
              }
              frame #2 {
                w99 = u8 0 ("Disabled")
                n223 = local write "ConnectChannel"(FALSE ("ConnectChannel")) -> ()
                n224 = property on="Quit" class="Bool (strict)"("Disabled"=w99) -> ()  [unwired: 2 in, 2 out]
                n225 = property on="Set Output OFF All" class="Bool (strict)"("Disabled"=w99) -> ()  [unwired: 2 in, 2 out]
                n226 = property on="ConnectAll" class="Bool (strict)"("Disabled"=w99) -> ()  [unwired: 2 in, 2 out]
                n227 = property on="Set Output ON All" class="Bool (strict)"("Disabled"=w99) -> ()  [unwired: 2 in, 2 out]
                n228 = property on="AddChannel" class="Bool (strict)"("Disabled"=w99) -> ()  [unwired: 2 in, 2 out]
                n229 = property on="DisconnectChannel" class="Bool (strict)"("Disabled"=w99) -> ()  [unwired: 2 in, 2 out]
                n230 = property on="ReadFromFile" class="Bool (strict)"("Disabled"=w99) -> ()  [unwired: 2 in, 2 out]
                n231 = property on="ConnectChannel" class="Bool (strict)"("Disabled"=w99) -> ()  [unwired: 2 in, 2 out]
                n232 = property on="DeleteChannel" class="Bool (strict)"("Disabled"=w99) -> ()  [unwired: 2 in, 2 out]
                n233 = property on="DisconnectAll" class="Bool (strict)"("Disabled"=w99) -> ()  [unwired: 2 in, 2 out]
                n234 = property on="CurrentModulationB" class="Bool (strict)"("Disabled"=w99) -> ()  [unwired: 2 in, 2 out]
                n235 = property on="WriteToFile" class="Bool (strict)"("Disabled"=w99) -> ()  [unwired: 2 in, 2 out]
                n236 = property on="SetCurrentB" class="Bool (strict)"("Disabled"=w99) -> ()  [unwired: 2 in, 2 out]
                n237 = property on="SetOutputOnB" class="Bool (strict)"("Disabled"=w99) -> ()  [unwired: 2 in, 2 out]
                n238 = property on="SetVoltageB" class="Bool (strict)"("Disabled"=w99) -> ()  [unwired: 2 in, 2 out]
                n239 = property on="SetOutputOffB" class="Bool (strict)"("Disabled"=w99) -> ()  [unwired: 2 in, 2 out]
                n240 = property on="SetVoltageAll" class="Bool (strict)"("Disabled"=w99) -> ()  [unwired: 2 in, 2 out]
                n241 = property on="SetCurrentAll" class="Bool (strict)"("Disabled"=w99) -> ()  [unwired: 2 in, 2 out]
              }
            }
          }
        }
      }
      event "ConnectAll": Value Change {
        n242 = event-data() -> ()  [unwired: 7 out]
        n243 = local read "ConnectAll"() -> (w101:bool)
        n244 = case shown="True" w101 {
          frame False {
            n245 = local write "ConnectAll"(FALSE ("ConnectChannel")) -> ()
          }
          frame True {
            n246 = flat-sequence {
              frame #0 {
                w119 = u8 2 ("Disabled")
                n247 = property on="ConnectChannel" class="Bool (strict)"("Disabled"=w119) -> (error out=w112:errorcluster)  [unwired: 2 in, 1 out]
                n248 = property on="Set Output OFF All" class="Bool (strict)"("Disabled"=w119) -> (error out=w118:errorcluster)  [unwired: 2 in, 1 out]
                n249 = property on="DeleteChannel" class="Bool (strict)"(error in=w112, "Disabled"=w119) -> (error out=w111:errorcluster)  [unwired: 1 in, 1 out]
                n250 = property on="ConnectAll" class="Bool (strict)"(error in=w118, "Disabled"=w119) -> (error out=w117:errorcluster)  [unwired: 1 in, 1 out]
                n251 = property on="Set Output ON All" class="Bool (strict)"(error in=w117, "Disabled"=w119) -> (error out=w116:errorcluster)  [unwired: 1 in, 1 out]
                n252 = property on="WriteToFile" class="Bool (strict)"(error in=w111, "Disabled"=w119) -> (error out=w110:errorcluster)  [unwired: 1 in, 1 out]
                n253 = property on="AddChannel" class="Bool (strict)"(error in=w116, "Disabled"=w119) -> (error out=w115:errorcluster)  [unwired: 1 in, 1 out]
                n254 = property on="SetCurrentB" class="Bool (strict)"(error in=w110, "Disabled"=w119) -> (error out=w109:errorcluster)  [unwired: 1 in, 1 out]
                n255 = property on="CurrentModulationB" class="Bool (strict)"(error in=w115, "Disabled"=w119) -> (error out=w114:errorcluster)  [unwired: 1 in, 1 out]
                n256 = property on="Quit" class="Bool (strict)"(error in=w109, "Disabled"=w119) -> (error out=w108:errorcluster)  [unwired: 1 in, 1 out]
                n257 = property on="SetOutputOnB" class="Bool (strict)"(error in=w108, "Disabled"=w119) -> (error out=w107:errorcluster)  [unwired: 1 in, 1 out]
                n258 = property on="DisconnectChannel" class="Bool (strict)"(error in=w114, "Disabled"=w119) -> (error out=w113:errorcluster)  [unwired: 1 in, 1 out]
                n259 = property on="SetVoltageB" class="Bool (strict)"(error in=w107, "Disabled"=w119) -> (error out=w106:errorcluster)  [unwired: 1 in, 1 out]
                n260 = property on="SetOutputOffB" class="Bool (strict)"(error in=w106, "Disabled"=w119) -> (error out=w105:errorcluster)  [unwired: 1 in, 1 out]
                n261 = property on="ReadFromFile" class="Bool (strict)"(error in=w113, "Disabled"=w119) -> ()  [unwired: 1 in, 2 out]
                n262 = property on="SetVoltageAll" class="Bool (strict)"(error in=w105, "Disabled"=w119) -> (error out=w104:errorcluster)  [unwired: 1 in, 1 out]
                n263 = property on="SetCurrentAll" class="Bool (strict)"(error in=w104, "Disabled"=w119) -> (error out=w103:errorcluster)  [unwired: 1 in, 1 out]
                n264 = property on="DisconnectAll" class="Bool (strict)"(error in=w103, "Disabled"=w119) -> ()  [unwired: 1 in, 2 out]
              }
              frame #1 {
                n265 = local read "VIRef"() -> (w121:refnum<vi>[])
                n266 = Array Size(array=w121) -> (size(s)=w120:i32)
                n267 = for {
                  N: w120 -> [_]
                  i -> [w122]
                  n268 = local read "VIRef"() -> (w125:refnum<vi>[])
                  n269 = Index Array(array=w125, index=w122) -> (element=w124:refnum<vi>)
                  n270 = invoke class="VI" method="Ctrl Val.Set"(reference=w124, "Control Name"="Connect", "Value"=TRUE ("OK Button")) -> ()  [unwired: 2 in, 5 out]
                }
              }
              frame #2 {
                w141 = u8 0 ("Disabled")
                n271 = local write "ConnectAll"(FALSE ("ConnectChannel")) -> ()
                n272 = property on="SetOutputOffB" class="Bool (strict)"("Disabled"=w141) -> (error out=w129:errorcluster)  [unwired: 2 in, 1 out]
                n273 = property on="ReadFromFile" class="Bool (strict)"("Disabled"=w141) -> (error out=w135:errorcluster)  [unwired: 2 in, 1 out]
                n274 = property on="Set Output OFF All" class="Bool (strict)"("Disabled"=w141) -> (error out=w140:errorcluster)  [unwired: 2 in, 1 out]
                n275 = property on="Quit" class="Bool (strict)"("Disabled"=w141) -> (error out=w131:errorcluster)  [unwired: 2 in, 1 out]
                n276 = property on="SetOutputOnB" class="Bool (strict)"(error in=w131, "Disabled"=w141) -> (error out=w130:errorcluster)  [unwired: 1 in, 1 out]
                n277 = property on="SetVoltageAll" class="Bool (strict)"(error in=w129, "Disabled"=w141) -> (error out=w128:errorcluster)  [unwired: 1 in, 1 out]
                n278 = property on="ConnectChannel" class="Bool (strict)"(error in=w135, "Disabled"=w141) -> (error out=w134:errorcluster)  [unwired: 1 in, 1 out]
                n279 = property on="ConnectAll" class="Bool (strict)"(error in=w140, "Disabled"=w141) -> (error out=w139:errorcluster)  [unwired: 1 in, 1 out]
                n280 = property on="SetCurrentAll" class="Bool (strict)"(error in=w128, "Disabled"=w141) -> (error out=w127:errorcluster)  [unwired: 1 in, 1 out]
                n281 = property on="SetVoltageB" class="Bool (strict)"(error in=w130, "Disabled"=w141) -> ()  [unwired: 1 in, 2 out]
                n282 = property on="Set Output ON All" class="Bool (strict)"(error in=w139, "Disabled"=w141) -> (error out=w138:errorcluster)  [unwired: 1 in, 1 out]
                n283 = property on="DisconnectAll" class="Bool (strict)"(error in=w127, "Disabled"=w141) -> ()  [unwired: 1 in, 2 out]
                n284 = property on="DeleteChannel" class="Bool (strict)"(error in=w134, "Disabled"=w141) -> (error out=w133:errorcluster)  [unwired: 1 in, 1 out]
                n285 = property on="AddChannel" class="Bool (strict)"(error in=w138, "Disabled"=w141) -> (error out=w137:errorcluster)  [unwired: 1 in, 1 out]
                n286 = property on="WriteToFile" class="Bool (strict)"(error in=w133, "Disabled"=w141) -> (error out=w132:errorcluster)  [unwired: 1 in, 1 out]
                n287 = property on="CurrentModulationB" class="Bool (strict)"(error in=w137, "Disabled"=w141) -> (error out=w136:errorcluster)  [unwired: 1 in, 1 out]
                n288 = property on="SetCurrentB" class="Bool (strict)"(error in=w132, "Disabled"=w141) -> ()  [unwired: 1 in, 2 out]
                n289 = property on="DisconnectChannel" class="Bool (strict)"(error in=w136, "Disabled"=w141) -> ()  [unwired: 1 in, 2 out]
              }
            }
          }
        }
      }
      event "DisconnectAll": Value Change {
        n290 = event-data() -> ()  [unwired: 7 out]
        n291 = local read "DisconnectAll"() -> (w143:bool)
        n292 = case shown="True" w143 {
          frame False {
            n293 = local write "DisconnectAll"(FALSE ("ConnectChannel")) -> ()
          }
          frame True {
            n294 = flat-sequence {
              frame #0 {
                w161 = u8 2 ("Disabled")
                n295 = property on="ConnectAll" class="Bool (strict)"("Disabled"=w161) -> (error out=w160:errorcluster)  [unwired: 2 in, 1 out]
                n296 = property on="DeleteChannel" class="Bool (strict)"("Disabled"=w161) -> (error out=w153:errorcluster)  [unwired: 2 in, 1 out]
                n297 = property on="Set Output OFF All" class="Bool (strict)"(error in=w160, "Disabled"=w161) -> (error out=w159:errorcluster)  [unwired: 1 in, 1 out]
                n298 = property on="WriteToFile" class="Bool (strict)"(error in=w153, "Disabled"=w161) -> (error out=w152:errorcluster)  [unwired: 1 in, 1 out]
                n299 = property on="AddChannel" class="Bool (strict)"(error in=w159, "Disabled"=w161) -> (error out=w158:errorcluster)  [unwired: 1 in, 1 out]
                n300 = property on="SetCurrentB" class="Bool (strict)"(error in=w152, "Disabled"=w161) -> (error out=w151:errorcluster)  [unwired: 1 in, 1 out]
                n301 = property on="Set Output ON All" class="Bool (strict)"(error in=w158, "Disabled"=w161) -> (error out=w157:errorcluster)  [unwired: 1 in, 1 out]
                n302 = property on="Quit" class="Bool (strict)"(error in=w151, "Disabled"=w161) -> (error out=w150:errorcluster)  [unwired: 1 in, 1 out]
                n303 = property on="SetOutputOnB" class="Bool (strict)"(error in=w150, "Disabled"=w161) -> (error out=w149:errorcluster)  [unwired: 1 in, 1 out]
                n304 = property on="CurrentModulationB" class="Bool (strict)"(error in=w157, "Disabled"=w161) -> (error out=w156:errorcluster)  [unwired: 1 in, 1 out]
                n305 = property on="SetVoltageB" class="Bool (strict)"(error in=w149, "Disabled"=w161) -> (error out=w148:errorcluster)  [unwired: 1 in, 1 out]
                n306 = property on="DisconnectChannel" class="Bool (strict)"(error in=w156, "Disabled"=w161) -> (error out=w155:errorcluster)  [unwired: 1 in, 1 out]
                n307 = property on="SetOutputOffB" class="Bool (strict)"(error in=w148, "Disabled"=w161) -> (error out=w147:errorcluster)  [unwired: 1 in, 1 out]
                n308 = property on="ReadFromFile" class="Bool (strict)"(error in=w155, "Disabled"=w161) -> (error out=w154:errorcluster)  [unwired: 1 in, 1 out]
                n309 = property on="SetVoltageAll" class="Bool (strict)"(error in=w147, "Disabled"=w161) -> (error out=w146:errorcluster)  [unwired: 1 in, 1 out]
                n310 = property on="SetCurrentAll" class="Bool (strict)"(error in=w146, "Disabled"=w161) -> (error out=w145:errorcluster)  [unwired: 1 in, 1 out]
                n311 = property on="ConnectChannel" class="Bool (strict)"(error in=w154, "Disabled"=w161) -> ()  [unwired: 1 in, 2 out]
                n312 = property on="DisconnectAll" class="Bool (strict)"(error in=w145, "Disabled"=w161) -> ()  [unwired: 1 in, 2 out]
              }
              frame #1 {
                n313 = local read "VIRef"() -> (w163:refnum<vi>[])
                n314 = Array Size(array=w163) -> (size(s)=w162:i32)
                n315 = for {
                  N: w162 -> [_]
                  i -> [w164]
                  n316 = local read "VIRef"() -> (w167:refnum<vi>[])
                  n317 = Index Array(array=w167, index=w164) -> (element=w166:refnum<vi>)
                  n318 = invoke class="VI" method="Ctrl Val.Set"(reference=w166, "Control Name"="Connect", "Value"=FALSE ("OK Button")) -> ()  [unwired: 2 in, 5 out]
                }
              }
              frame #2 {
                w184 = u8 0 ("Disabled")
                n319 = local write "DisconnectAll"(FALSE ("ConnectChannel")) -> ()
                n320 = property on="Set Output OFF All" class="Bool (strict)"("Disabled"=w184) -> (error out=w183:errorcluster)  [unwired: 2 in, 1 out]
                n321 = property on="DeleteChannel" class="Bool (strict)"("Disabled"=w184) -> (error out=w176:errorcluster)  [unwired: 2 in, 1 out]
                n322 = property on="SetCurrentB" class="Bool (strict)"("Disabled"=w184) -> (error out=w175:errorcluster)  [unwired: 2 in, 1 out]
                n323 = property on="Quit" class="Bool (strict)"(error in=w175, "Disabled"=w184) -> (error out=w174:errorcluster)  [unwired: 1 in, 1 out]
                n324 = property on="WriteToFile" class="Bool (strict)"(error in=w176, "Disabled"=w184) -> ()  [unwired: 1 in, 2 out]
                n325 = property on="SetOutputOnB" class="Bool (strict)"(error in=w174, "Disabled"=w184) -> (error out=w173:errorcluster)  [unwired: 1 in, 1 out]
                n326 = property on="ConnectAll" class="Bool (strict)"(error in=w183, "Disabled"=w184) -> (error out=w182:errorcluster)  [unwired: 1 in, 1 out]
                n327 = property on="Set Output ON All" class="Bool (strict)"(error in=w182, "Disabled"=w184) -> (error out=w181:errorcluster)  [unwired: 1 in, 1 out]
                n328 = property on="SetVoltageB" class="Bool (strict)"(error in=w173, "Disabled"=w184) -> (error out=w172:errorcluster)  [unwired: 1 in, 1 out]
                n329 = property on="AddChannel" class="Bool (strict)"(error in=w181, "Disabled"=w184) -> (error out=w180:errorcluster)  [unwired: 1 in, 1 out]
                n330 = property on="SetOutputOffB" class="Bool (strict)"(error in=w172, "Disabled"=w184) -> (error out=w171:errorcluster)  [unwired: 1 in, 1 out]
                n331 = property on="CurrentModulationB" class="Bool (strict)"(error in=w180, "Disabled"=w184) -> (error out=w179:errorcluster)  [unwired: 1 in, 1 out]
                n332 = property on="SetVoltageAll" class="Bool (strict)"(error in=w171, "Disabled"=w184) -> (error out=w170:errorcluster)  [unwired: 1 in, 1 out]
                n333 = property on="DisconnectChannel" class="Bool (strict)"(error in=w179, "Disabled"=w184) -> (error out=w178:errorcluster)  [unwired: 1 in, 1 out]
                n334 = property on="SetCurrentAll" class="Bool (strict)"(error in=w170, "Disabled"=w184) -> (error out=w169:errorcluster)  [unwired: 1 in, 1 out]
                n335 = property on="DisconnectAll" class="Bool (strict)"(error in=w169, "Disabled"=w184) -> ()  [unwired: 1 in, 2 out]
                n336 = property on="ReadFromFile" class="Bool (strict)"(error in=w178, "Disabled"=w184) -> (error out=w177:errorcluster)  [unwired: 1 in, 1 out]
                n337 = property on="ConnectChannel" class="Bool (strict)"(error in=w177, "Disabled"=w184) -> ()  [unwired: 1 in, 2 out]
              }
            }
          }
        }
      }
      event "SetVoltageB": Value Change {
        n338 = event-data() -> ()  [unwired: 7 out]
        n339 = property on="List of channels" class="MCListbox (strict)"() -> ("Value"=w186:i32)  [unwired: 2 in, 2 out]
        n340 = local read "SetVoltageB"() -> (w187:bool)
        n341 = Greater Or Equal?(x=w186, y=0) -> (x >= y?=w189:bool)
        n342 = And(x=w189, y=w187) -> (x .and. y?=w188:bool)
        n343 = case shown="True" w188 {
          tunnel: w186 -> [_ w192]
          frame False {
            n344 = local write "SetVoltageB"(FALSE ("ConnectChannel")) -> ()
          }
          frame True {
            n345 = flat-sequence {
              tunnel: w192 -> [w199]
              frame #0 {
                w194 = u8 2 ("Disabled")
                n346 = property on="Quit" class="Bool (strict)"("Disabled"=w194) -> ()  [unwired: 2 in, 2 out]
                n347 = property on="ConnectAll" class="Bool (strict)"("Disabled"=w194) -> ()  [unwired: 2 in, 2 out]
                n348 = property on="Set Output OFF All" class="Bool (strict)"("Disabled"=w194) -> ()  [unwired: 2 in, 2 out]
                n349 = property on="AddChannel" class="Bool (strict)"("Disabled"=w194) -> ()  [unwired: 2 in, 2 out]
                n350 = property on="Set Output ON All" class="Bool (strict)"("Disabled"=w194) -> ()  [unwired: 2 in, 2 out]
                n351 = property on="CurrentModulationB" class="Bool (strict)"("Disabled"=w194) -> ()  [unwired: 2 in, 2 out]
                n352 = property on="DisconnectChannel" class="Bool (strict)"("Disabled"=w194) -> ()  [unwired: 2 in, 2 out]
                n353 = property on="ReadFromFile" class="Bool (strict)"("Disabled"=w194) -> ()  [unwired: 2 in, 2 out]
                n354 = property on="ConnectChannel" class="Bool (strict)"("Disabled"=w194) -> ()  [unwired: 2 in, 2 out]
                n355 = property on="DeleteChannel" class="Bool (strict)"("Disabled"=w194) -> ()  [unwired: 2 in, 2 out]
                n356 = property on="WriteToFile" class="Bool (strict)"("Disabled"=w194) -> ()  [unwired: 2 in, 2 out]
                n357 = property on="SetCurrentB" class="Bool (strict)"("Disabled"=w194) -> ()  [unwired: 2 in, 2 out]
                n358 = property on="SetOutputOnB" class="Bool (strict)"("Disabled"=w194) -> ()  [unwired: 2 in, 2 out]
                n359 = property on="SetVoltageB" class="Bool (strict)"("Disabled"=w194) -> ()  [unwired: 2 in, 2 out]
                n360 = property on="SetOutputOffB" class="Bool (strict)"("Disabled"=w194) -> ()  [unwired: 2 in, 2 out]
                n361 = property on="SetVoltageAll" class="Bool (strict)"("Disabled"=w194) -> ()  [unwired: 2 in, 2 out]
                n362 = property on="SetCurrentAll" class="Bool (strict)"("Disabled"=w194) -> ()  [unwired: 2 in, 2 out]
                n363 = property on="DisconnectAll" class="Bool (strict)"("Disabled"=w194) -> ()  [unwired: 2 in, 2 out]
              }
              frame #1 {
                n364 = local read "VIRef"() -> (w201:refnum<vi>[])
                n365 = local read "SetVoltage"() -> (w198:dbl)
                n366 = Index Array(array=w201, index=w199) -> (element=w200:refnum<vi>)
                n367 = invoke class="VI" method="Ctrl Val.Set"(reference=w200, "Control Name"="SetVoltage", "Value"=w198) -> (reference out=w195:refnum<vi>)  [unwired: 2 in, 4 out]
                n368 = invoke class="VI" method="Ctrl Val.Set"(reference=w195, "Control Name"="NeedToSetVoltage", "Value"=TRUE ("ConnectChannel")) -> ()  [unwired: 2 in, 5 out]
              }
              frame #2 {
                w203 = u8 0 ("Disabled")
                n369 = property on="Quit" class="Bool (strict)"("Disabled"=w203) -> ()  [unwired: 2 in, 2 out]
                n370 = property on="Set Output OFF All" class="Bool (strict)"("Disabled"=w203) -> ()  [unwired: 2 in, 2 out]
                n371 = property on="ConnectAll" class="Bool (strict)"("Disabled"=w203) -> ()  [unwired: 2 in, 2 out]
                n372 = property on="Set Output ON All" class="Bool (strict)"("Disabled"=w203) -> ()  [unwired: 2 in, 2 out]
                n373 = property on="AddChannel" class="Bool (strict)"("Disabled"=w203) -> ()  [unwired: 2 in, 2 out]
                n374 = property on="CurrentModulationB" class="Bool (strict)"("Disabled"=w203) -> ()  [unwired: 2 in, 2 out]
                n375 = property on="DisconnectChannel" class="Bool (strict)"("Disabled"=w203) -> ()  [unwired: 2 in, 2 out]
                n376 = property on="ReadFromFile" class="Bool (strict)"("Disabled"=w203) -> ()  [unwired: 2 in, 2 out]
                n377 = property on="ConnectChannel" class="Bool (strict)"("Disabled"=w203) -> ()  [unwired: 2 in, 2 out]
                n378 = property on="DeleteChannel" class="Bool (strict)"("Disabled"=w203) -> ()  [unwired: 2 in, 2 out]
                n379 = property on="WriteToFile" class="Bool (strict)"("Disabled"=w203) -> ()  [unwired: 2 in, 2 out]
                n380 = property on="SetCurrentB" class="Bool (strict)"("Disabled"=w203) -> ()  [unwired: 2 in, 2 out]
                n381 = property on="SetOutputOnB" class="Bool (strict)"("Disabled"=w203) -> ()  [unwired: 2 in, 2 out]
                n382 = property on="SetVoltageB" class="Bool (strict)"("Disabled"=w203) -> ()  [unwired: 2 in, 2 out]
                n383 = property on="SetOutputOffB" class="Bool (strict)"("Disabled"=w203) -> ()  [unwired: 2 in, 2 out]
                n384 = property on="SetVoltageAll" class="Bool (strict)"("Disabled"=w203) -> ()  [unwired: 2 in, 2 out]
                n385 = property on="SetCurrentAll" class="Bool (strict)"("Disabled"=w203) -> ()  [unwired: 2 in, 2 out]
                n386 = property on="DisconnectAll" class="Bool (strict)"("Disabled"=w203) -> ()  [unwired: 2 in, 2 out]
              }
            }
            n387 = local write "SetVoltageB"(FALSE ("ConnectChannel")) -> ()
          }
        }
      }
      event "SetOutputOnB": Value Change {
        n388 = event-data() -> ()  [unwired: 7 out]
        n389 = property on="List of channels" class="MCListbox (strict)"() -> ("Value"=w204:i32)  [unwired: 2 in, 2 out]
        n390 = local read "SetOutputOnB"() -> (w205:bool)
        n391 = Greater Or Equal?(x=w204, y=0) -> (x >= y?=w207:bool)
        n392 = And(x=w207, y=w205) -> (x .and. y?=w206:bool)
        n393 = case shown="True" w206 {
          tunnel: w204 -> [_ w211]
          frame False {
            n394 = local write "SetOutputOnB"(FALSE ("ConnectChannel")) -> ()
          }
          frame True {
            n395 = flat-sequence {
              tunnel: w211 -> [w213]
              tunnel: [w213] -> w210
              tunnel: w210 -> [w218]
              frame #0 {
                w212 = u8 2 ("Disabled")
                n396 = property on="Quit" class="Bool (strict)"("Disabled"=w212) -> ()  [unwired: 2 in, 2 out]
                n397 = property on="Set Output OFF All" class="Bool (strict)"("Disabled"=w212) -> ()  [unwired: 2 in, 2 out]
                n398 = property on="ConnectAll" class="Bool (strict)"("Disabled"=w212) -> ()  [unwired: 2 in, 2 out]
                n399 = property on="Set Output ON All" class="Bool (strict)"("Disabled"=w212) -> ()  [unwired: 2 in, 2 out]
                n400 = property on="AddChannel" class="Bool (strict)"("Disabled"=w212) -> ()  [unwired: 2 in, 2 out]
                n401 = property on="CurrentModulationB" class="Bool (strict)"("Disabled"=w212) -> ()  [unwired: 2 in, 2 out]
                n402 = property on="DisconnectChannel" class="Bool (strict)"("Disabled"=w212) -> ()  [unwired: 2 in, 2 out]
                n403 = property on="ReadFromFile" class="Bool (strict)"("Disabled"=w212) -> ()  [unwired: 2 in, 2 out]
                n404 = property on="ConnectChannel" class="Bool (strict)"("Disabled"=w212) -> ()  [unwired: 2 in, 2 out]
                n405 = property on="DeleteChannel" class="Bool (strict)"("Disabled"=w212) -> ()  [unwired: 2 in, 2 out]
                n406 = property on="WriteToFile" class="Bool (strict)"("Disabled"=w212) -> ()  [unwired: 2 in, 2 out]
                n407 = property on="SetCurrentB" class="Bool (strict)"("Disabled"=w212) -> ()  [unwired: 2 in, 2 out]
                n408 = property on="SetOutputOnB" class="Bool (strict)"("Disabled"=w212) -> ()  [unwired: 2 in, 2 out]
                n409 = property on="SetVoltageB" class="Bool (strict)"("Disabled"=w212) -> ()  [unwired: 2 in, 2 out]
                n410 = property on="SetOutputOffB" class="Bool (strict)"("Disabled"=w212) -> ()  [unwired: 2 in, 2 out]
                n411 = property on="SetVoltageAll" class="Bool (strict)"("Disabled"=w212) -> ()  [unwired: 2 in, 2 out]
                n412 = property on="SetCurrentAll" class="Bool (strict)"("Disabled"=w212) -> ()  [unwired: 2 in, 2 out]
                n413 = property on="DisconnectAll" class="Bool (strict)"("Disabled"=w212) -> ()  [unwired: 2 in, 2 out]
              }
              frame #1 {
                n414 = local read "VIRef"() -> (w221:refnum<vi>[])
                n415 = local write "SetOutputOnB"(FALSE ("ConnectChannel")) -> ()
                n416 = Index Array(array=w221, index=w218) -> (element=w220:refnum<vi>)
                n417 = invoke class="VI" method="Ctrl Val.Set"(reference=w220, "Control Name"="SetOutput", "Value"=TRUE ("ConnectChannel")) -> (reference out=w215:refnum<vi>)  [unwired: 2 in, 4 out]
                n418 = invoke class="VI" method="Ctrl Val.Set"(reference=w215, "Control Name"="NeedToSetOutput", "Value"=TRUE ("ConnectChannel")) -> ()  [unwired: 2 in, 5 out]
              }
              frame #2 {
                w223 = u8 0 ("Disabled")
                n419 = property on="Quit" class="Bool (strict)"("Disabled"=w223) -> ()  [unwired: 2 in, 2 out]
                n420 = property on="Set Output OFF All" class="Bool (strict)"("Disabled"=w223) -> ()  [unwired: 2 in, 2 out]
                n421 = property on="ConnectAll" class="Bool (strict)"("Disabled"=w223) -> ()  [unwired: 2 in, 2 out]
                n422 = property on="Set Output ON All" class="Bool (strict)"("Disabled"=w223) -> ()  [unwired: 2 in, 2 out]
                n423 = property on="AddChannel" class="Bool (strict)"("Disabled"=w223) -> ()  [unwired: 2 in, 2 out]
                n424 = property on="DisconnectChannel" class="Bool (strict)"("Disabled"=w223) -> ()  [unwired: 2 in, 2 out]
                n425 = property on="ReadFromFile" class="Bool (strict)"("Disabled"=w223) -> ()  [unwired: 2 in, 2 out]
                n426 = property on="ConnectChannel" class="Bool (strict)"("Disabled"=w223) -> ()  [unwired: 2 in, 2 out]
                n427 = property on="DeleteChannel" class="Bool (strict)"("Disabled"=w223) -> ()  [unwired: 2 in, 2 out]
                n428 = property on="SetOutputOffB" class="Bool (strict)"("Disabled"=w223) -> ()  [unwired: 2 in, 2 out]
                n429 = property on="CurrentModulationB" class="Bool (strict)"("Disabled"=w223) -> ()  [unwired: 2 in, 2 out]
                n430 = property on="SetVoltageAll" class="Bool (strict)"("Disabled"=w223) -> ()  [unwired: 2 in, 2 out]
                n431 = property on="SetCurrentAll" class="Bool (strict)"("Disabled"=w223) -> ()  [unwired: 2 in, 2 out]
                n432 = property on="DisconnectAll" class="Bool (strict)"("Disabled"=w223) -> ()  [unwired: 2 in, 2 out]
                n433 = property on="WriteToFile" class="Bool (strict)"("Disabled"=w223) -> ()  [unwired: 2 in, 2 out]
                n434 = property on="SetCurrentB" class="Bool (strict)"("Disabled"=w223) -> ()  [unwired: 2 in, 2 out]
                n435 = property on="SetOutputOnB" class="Bool (strict)"("Disabled"=w223) -> ()  [unwired: 2 in, 2 out]
                n436 = property on="SetVoltageB" class="Bool (strict)"("Disabled"=w223) -> ()  [unwired: 2 in, 2 out]
              }
            }
          }
        }
      }
      event "Set Output ON All": Value Change {
        n437 = event-data() -> ()  [unwired: 7 out]
        n438 = local read "Set Output ON All"() -> (w224:bool)
        n439 = case shown="True" w224 {
          frame False {
            n440 = local write "Set Output ON All"(FALSE ("ConnectChannel")) -> ()
          }
          frame True {
            n441 = flat-sequence {
              frame #0 {
                w226 = u8 2 ("Disabled")
                n442 = property on="Quit" class="Bool (strict)"("Disabled"=w226) -> ()  [unwired: 2 in, 2 out]
                n443 = property on="AddChannel" class="Bool (strict)"("Disabled"=w226) -> ()  [unwired: 2 in, 2 out]
                n444 = property on="CurrentModulationB" class="Bool (strict)"("Disabled"=w226) -> ()  [unwired: 2 in, 2 out]
                n445 = property on="DisconnectChannel" class="Bool (strict)"("Disabled"=w226) -> ()  [unwired: 2 in, 2 out]
                n446 = property on="ConnectAll" class="Bool (strict)"("Disabled"=w226) -> ()  [unwired: 2 in, 2 out]
                n447 = property on="ReadFromFile" class="Bool (strict)"("Disabled"=w226) -> ()  [unwired: 2 in, 2 out]
                n448 = property on="ConnectChannel" class="Bool (strict)"("Disabled"=w226) -> ()  [unwired: 2 in, 2 out]
                n449 = property on="DeleteChannel" class="Bool (strict)"("Disabled"=w226) -> ()  [unwired: 2 in, 2 out]
                n450 = property on="WriteToFile" class="Bool (strict)"("Disabled"=w226) -> ()  [unwired: 2 in, 2 out]
                n451 = property on="SetCurrentB" class="Bool (strict)"("Disabled"=w226) -> ()  [unwired: 2 in, 2 out]
                n452 = property on="SetOutputOnB" class="Bool (strict)"("Disabled"=w226) -> ()  [unwired: 2 in, 2 out]
                n453 = property on="SetVoltageB" class="Bool (strict)"("Disabled"=w226) -> ()  [unwired: 2 in, 2 out]
                n454 = property on="SetOutputOffB" class="Bool (strict)"("Disabled"=w226) -> ()  [unwired: 2 in, 2 out]
                n455 = property on="SetVoltageAll" class="Bool (strict)"("Disabled"=w226) -> ()  [unwired: 2 in, 2 out]
                n456 = property on="SetCurrentAll" class="Bool (strict)"("Disabled"=w226) -> ()  [unwired: 2 in, 2 out]
                n457 = property on="DisconnectAll" class="Bool (strict)"("Disabled"=w226) -> ()  [unwired: 2 in, 2 out]
              }
              frame #1 {
                n458 = local read "VIRef"() -> (w228:refnum<vi>[])
                n459 = Array Size(array=w228) -> (size(s)=w227:i32)
                n460 = for {
                  N: w227 -> [_]
                  i -> [w229]
                  n461 = local read "VIRef"() -> (w235:refnum<vi>[])
                  n462 = Index Array(array=w235, index=w229) -> (element=w234:refnum<vi>)
                  n463 = invoke class="VI" method="Ctrl Val.Set"(reference=w234, "Control Name"="SetOutput", "Value"=TRUE ("ConnectChannel")) -> (reference out=w231:refnum<vi>)  [unwired: 2 in, 4 out]
                  n464 = invoke class="VI" method="Ctrl Val.Set"(reference=w231, "Control Name"="NeedToSetOutput", "Value"=TRUE ("ConnectChannel")) -> ()  [unwired: 2 in, 5 out]
                }
              }
              frame #2 {
                w237 = u8 0 ("Disabled")
                n465 = local write "Set Output ON All"(FALSE ("ConnectChannel")) -> ()
                n466 = property on="Quit" class="Bool (strict)"("Disabled"=w237) -> ()  [unwired: 2 in, 2 out]
                n467 = property on="Set Output OFF All" class="Bool (strict)"("Disabled"=w237) -> ()  [unwired: 2 in, 2 out]
                n468 = property on="ConnectAll" class="Bool (strict)"("Disabled"=w237) -> ()  [unwired: 2 in, 2 out]
                n469 = property on="Set Output ON All" class="Bool (strict)"("Disabled"=w237) -> ()  [unwired: 2 in, 2 out]
                n470 = property on="AddChannel" class="Bool (strict)"("Disabled"=w237) -> ()  [unwired: 2 in, 2 out]
                n471 = property on="DisconnectChannel" class="Bool (strict)"("Disabled"=w237) -> ()  [unwired: 2 in, 2 out]
                n472 = property on="ReadFromFile" class="Bool (strict)"("Disabled"=w237) -> ()  [unwired: 2 in, 2 out]
                n473 = property on="ConnectChannel" class="Bool (strict)"("Disabled"=w237) -> ()  [unwired: 2 in, 2 out]
                n474 = property on="DeleteChannel" class="Bool (strict)"("Disabled"=w237) -> ()  [unwired: 2 in, 2 out]
                n475 = property on="SetOutputOffB" class="Bool (strict)"("Disabled"=w237) -> ()  [unwired: 2 in, 2 out]
                n476 = property on="CurrentModulationB" class="Bool (strict)"("Disabled"=w237) -> ()  [unwired: 2 in, 2 out]
                n477 = property on="SetVoltageAll" class="Bool (strict)"("Disabled"=w237) -> ()  [unwired: 2 in, 2 out]
                n478 = property on="SetCurrentAll" class="Bool (strict)"("Disabled"=w237) -> ()  [unwired: 2 in, 2 out]
                n479 = property on="DisconnectAll" class="Bool (strict)"("Disabled"=w237) -> ()  [unwired: 2 in, 2 out]
                n480 = property on="WriteToFile" class="Bool (strict)"("Disabled"=w237) -> ()  [unwired: 2 in, 2 out]
                n481 = property on="SetCurrentB" class="Bool (strict)"("Disabled"=w237) -> ()  [unwired: 2 in, 2 out]
                n482 = property on="SetOutputOnB" class="Bool (strict)"("Disabled"=w237) -> ()  [unwired: 2 in, 2 out]
                n483 = property on="SetVoltageB" class="Bool (strict)"("Disabled"=w237) -> ()  [unwired: 2 in, 2 out]
              }
            }
          }
        }
      }
      event "SetOutputOffB": Value Change {
        n484 = event-data() -> ()  [unwired: 7 out]
        n485 = property on="List of channels" class="MCListbox (strict)"() -> ("Value"=w239:i32)  [unwired: 2 in, 2 out]
        n486 = local read "SetOutputOffB"() -> (w240:bool)
        n487 = Greater Or Equal?(x=w239, y=0) -> (x >= y?=w242:bool)
        n488 = And(x=w242, y=w240) -> (x .and. y?=w241:bool)
        n489 = case shown="True" w241 {
          tunnel: w239 -> [_ w247]
          frame False {
            n490 = local write "SetOutputOffB"(FALSE ("SetOutputOffB")) -> ()
          }
          frame True {
            n491 = flat-sequence {
              tunnel: w247 -> [w249]
              tunnel: [w249] -> w245
              tunnel: w245 -> [w254]
              frame #0 {
                w248 = u8 2 ("Disabled")
                n492 = property on="Quit" class="Bool (strict)"("Disabled"=w248) -> ()  [unwired: 2 in, 2 out]
                n493 = property on="Set Output OFF All" class="Bool (strict)"("Disabled"=w248) -> ()  [unwired: 2 in, 2 out]
                n494 = property on="ConnectAll" class="Bool (strict)"("Disabled"=w248) -> ()  [unwired: 2 in, 2 out]
                n495 = property on="Set Output ON All" class="Bool (strict)"("Disabled"=w248) -> ()  [unwired: 2 in, 2 out]
                n496 = property on="AddChannel" class="Bool (strict)"("Disabled"=w248) -> ()  [unwired: 2 in, 2 out]
                n497 = property on="CurrentModulationB" class="Bool (strict)"("Disabled"=w248) -> ()  [unwired: 2 in, 2 out]
                n498 = property on="DisconnectChannel" class="Bool (strict)"("Disabled"=w248) -> ()  [unwired: 2 in, 2 out]
                n499 = property on="ReadFromFile" class="Bool (strict)"("Disabled"=w248) -> ()  [unwired: 2 in, 2 out]
                n500 = property on="ConnectChannel" class="Bool (strict)"("Disabled"=w248) -> ()  [unwired: 2 in, 2 out]
                n501 = property on="DeleteChannel" class="Bool (strict)"("Disabled"=w248) -> ()  [unwired: 2 in, 2 out]
                n502 = property on="WriteToFile" class="Bool (strict)"("Disabled"=w248) -> ()  [unwired: 2 in, 2 out]
                n503 = property on="SetCurrentB" class="Bool (strict)"("Disabled"=w248) -> ()  [unwired: 2 in, 2 out]
                n504 = property on="SetOutputOnB" class="Bool (strict)"("Disabled"=w248) -> ()  [unwired: 2 in, 2 out]
                n505 = property on="SetVoltageB" class="Bool (strict)"("Disabled"=w248) -> ()  [unwired: 2 in, 2 out]
                n506 = property on="SetOutputOffB" class="Bool (strict)"("Disabled"=w248) -> ()  [unwired: 2 in, 2 out]
                n507 = property on="SetVoltageAll" class="Bool (strict)"("Disabled"=w248) -> ()  [unwired: 2 in, 2 out]
                n508 = property on="SetCurrentAll" class="Bool (strict)"("Disabled"=w248) -> ()  [unwired: 2 in, 2 out]
                n509 = property on="DisconnectAll" class="Bool (strict)"("Disabled"=w248) -> ()  [unwired: 2 in, 2 out]
              }
              frame #1 {
                n510 = local read "VIRef"() -> (w256:refnum<vi>[])
                n511 = Index Array(array=w256, index=w254) -> (element=w255:refnum<vi>)
                n512 = invoke class="VI" method="Ctrl Val.Set"(reference=w255, "Control Name"="SetOutput", "Value"=FALSE ("ConnectChannel")) -> (reference out=w251:refnum<vi>)  [unwired: 2 in, 4 out]
                n513 = invoke class="VI" method="Ctrl Val.Set"(reference=w251, "Control Name"="NeedToSetOutput", "Value"=TRUE ("ConnectChannel")) -> ()  [unwired: 2 in, 5 out]
              }
              frame #2 {
                w258 = u8 0 ("Disabled")
                n514 = property on="Quit" class="Bool (strict)"("Disabled"=w258) -> ()  [unwired: 2 in, 2 out]
                n515 = property on="ConnectAll" class="Bool (strict)"("Disabled"=w258) -> ()  [unwired: 2 in, 2 out]
                n516 = property on="Set Output ON All" class="Bool (strict)"("Disabled"=w258) -> ()  [unwired: 2 in, 2 out]
                n517 = property on="AddChannel" class="Bool (strict)"("Disabled"=w258) -> ()  [unwired: 2 in, 2 out]
                n518 = property on="CurrentModulationB" class="Bool (strict)"("Disabled"=w258) -> ()  [unwired: 2 in, 2 out]
                n519 = property on="DisconnectChannel" class="Bool (strict)"("Disabled"=w258) -> ()  [unwired: 2 in, 2 out]
                n520 = property on="ReadFromFile" class="Bool (strict)"("Disabled"=w258) -> ()  [unwired: 2 in, 2 out]
                n521 = property on="ConnectChannel" class="Bool (strict)"("Disabled"=w258) -> ()  [unwired: 2 in, 2 out]
                n522 = property on="DeleteChannel" class="Bool (strict)"("Disabled"=w258) -> ()  [unwired: 2 in, 2 out]
                n523 = property on="SetOutputOffB" class="Bool (strict)"("Disabled"=w258) -> ()  [unwired: 2 in, 2 out]
                n524 = property on="Set Output OFF All" class="Bool (strict)"("Disabled"=w258) -> ()  [unwired: 2 in, 2 out]
                n525 = property on="SetVoltageAll" class="Bool (strict)"("Disabled"=w258) -> ()  [unwired: 2 in, 2 out]
                n526 = property on="SetCurrentAll" class="Bool (strict)"("Disabled"=w258) -> ()  [unwired: 2 in, 2 out]
                n527 = property on="DisconnectAll" class="Bool (strict)"("Disabled"=w258) -> ()  [unwired: 2 in, 2 out]
                n528 = property on="WriteToFile" class="Bool (strict)"("Disabled"=w258) -> ()  [unwired: 2 in, 2 out]
                n529 = property on="SetCurrentB" class="Bool (strict)"("Disabled"=w258) -> ()  [unwired: 2 in, 2 out]
                n530 = property on="SetOutputOnB" class="Bool (strict)"("Disabled"=w258) -> ()  [unwired: 2 in, 2 out]
                n531 = property on="SetVoltageB" class="Bool (strict)"("Disabled"=w258) -> ()  [unwired: 2 in, 2 out]
              }
            }
            n532 = local write "SetOutputOffB"(FALSE ("ConnectChannel")) -> ()
          }
        }
      }
      event "Set Output OFF All": Value Change {
        n533 = event-data() -> ()  [unwired: 7 out]
        n534 = local read "Set Output OFF All"() -> (w259:bool)
        n535 = case shown="True" w259 {
          frame False {
            n536 = local write "Set Output OFF All"(FALSE ("SetOutputOffB")) -> ()
          }
          frame True {
            n537 = flat-sequence {
              frame #0 {
                w262 = u8 2 ("Disabled")
                n538 = property on="Quit" class="Bool (strict)"("Disabled"=w262) -> ()  [unwired: 2 in, 2 out]
                n539 = property on="ConnectAll" class="Bool (strict)"("Disabled"=w262) -> ()  [unwired: 2 in, 2 out]
                n540 = property on="Set Output OFF All" class="Bool (strict)"("Disabled"=w262) -> ()  [unwired: 2 in, 2 out]
                n541 = property on="AddChannel" class="Bool (strict)"("Disabled"=w262) -> ()  [unwired: 2 in, 2 out]
                n542 = property on="Set Output ON All" class="Bool (strict)"("Disabled"=w262) -> ()  [unwired: 2 in, 2 out]
                n543 = property on="CurrentModulationB" class="Bool (strict)"("Disabled"=w262) -> ()  [unwired: 2 in, 2 out]
                n544 = property on="DisconnectChannel" class="Bool (strict)"("Disabled"=w262) -> ()  [unwired: 2 in, 2 out]
                n545 = property on="ReadFromFile" class="Bool (strict)"("Disabled"=w262) -> ()  [unwired: 2 in, 2 out]
                n546 = property on="SetVoltageAll" class="Bool (strict)"("Disabled"=w262) -> ()  [unwired: 2 in, 2 out]
                n547 = property on="Set Output OFF All" class="Bool (strict)"("Disabled"=w262) -> ()  [unwired: 2 in, 2 out]
                n548 = property on="SetCurrentAll" class="Bool (strict)"("Disabled"=w262) -> ()  [unwired: 2 in, 2 out]
                n549 = property on="ConnectChannel" class="Bool (strict)"("Disabled"=w262) -> ()  [unwired: 2 in, 2 out]
                n550 = property on="DeleteChannel" class="Bool (strict)"("Disabled"=w262) -> ()  [unwired: 2 in, 2 out]
                n551 = property on="Set Output ON All" class="Bool (strict)"("Disabled"=w262) -> ()  [unwired: 2 in, 2 out]
                n552 = property on="DisconnectAll" class="Bool (strict)"("Disabled"=w262) -> ()  [unwired: 2 in, 2 out]
                n553 = property on="WriteToFile" class="Bool (strict)"("Disabled"=w262) -> ()  [unwired: 2 in, 2 out]
                n554 = property on="SetCurrentB" class="Bool (strict)"("Disabled"=w262) -> ()  [unwired: 2 in, 2 out]
                n555 = property on="SetOutputOnB" class="Bool (strict)"("Disabled"=w262) -> ()  [unwired: 2 in, 2 out]
                n556 = property on="SetVoltageB" class="Bool (strict)"("Disabled"=w262) -> ()  [unwired: 2 in, 2 out]
                n557 = property on="SetOutputOffB" class="Bool (strict)"("Disabled"=w262) -> ()  [unwired: 2 in, 2 out]
              }
              frame #1 {
                n558 = local read "VIRef"() -> (w263:refnum<vi>[])
                n559 = Array Size(array=w263) -> (size(s)=w264:i32)
                n560 = for {
                  N: w264 -> [_]
                  i -> [w265]
                  n561 = local read "VIRef"() -> (w271:refnum<vi>[])
                  n562 = Index Array(array=w271, index=w265) -> (element=w270:refnum<vi>)
                  n563 = invoke class="VI" method="Ctrl Val.Set"(reference=w270, "Control Name"="SetOutput", "Value"=FALSE ("ConnectChannel")) -> (reference out=w267:refnum<vi>)  [unwired: 2 in, 4 out]
                  n564 = invoke class="VI" method="Ctrl Val.Set"(reference=w267, "Control Name"="NeedToSetOutput", "Value"=TRUE ("ConnectChannel")) -> ()  [unwired: 2 in, 5 out]
                }
              }
              frame #2 {
                w273 = u8 0 ("Disabled")
                n565 = property on="Quit" class="Bool (strict)"("Disabled"=w273) -> ()  [unwired: 2 in, 2 out]
                n566 = property on="ConnectAll" class="Bool (strict)"("Disabled"=w273) -> ()  [unwired: 2 in, 2 out]
                n567 = property on="Set Output OFF All" class="Bool (strict)"("Disabled"=w273) -> ()  [unwired: 2 in, 2 out]
                n568 = property on="AddChannel" class="Bool (strict)"("Disabled"=w273) -> ()  [unwired: 2 in, 2 out]
                n569 = property on="CurrentModulationB" class="Bool (strict)"("Disabled"=w273) -> ()  [unwired: 2 in, 2 out]
                n570 = property on="DisconnectChannel" class="Bool (strict)"("Disabled"=w273) -> ()  [unwired: 2 in, 2 out]
                n571 = property on="ReadFromFile" class="Bool (strict)"("Disabled"=w273) -> ()  [unwired: 2 in, 2 out]
                n572 = property on="SetVoltageAll" class="Bool (strict)"("Disabled"=w273) -> ()  [unwired: 2 in, 2 out]
                n573 = property on="Set Output OFF All" class="Bool (strict)"("Disabled"=w273) -> ()  [unwired: 2 in, 2 out]
                n574 = property on="SetCurrentAll" class="Bool (strict)"("Disabled"=w273) -> ()  [unwired: 2 in, 2 out]
                n575 = property on="ConnectChannel" class="Bool (strict)"("Disabled"=w273) -> ()  [unwired: 2 in, 2 out]
                n576 = property on="DeleteChannel" class="Bool (strict)"("Disabled"=w273) -> ()  [unwired: 2 in, 2 out]
                n577 = property on="Set Output ON All" class="Bool (strict)"("Disabled"=w273) -> ()  [unwired: 2 in, 2 out]
                n578 = property on="DisconnectAll" class="Bool (strict)"("Disabled"=w273) -> ()  [unwired: 2 in, 2 out]
                n579 = property on="SetCurrentB" class="Bool (strict)"("Disabled"=w273) -> ()  [unwired: 2 in, 2 out]
                n580 = property on="Set Output ON All" class="Bool (strict)"("Disabled"=w273) -> ()  [unwired: 2 in, 2 out]
                n581 = property on="SetOutputOnB" class="Bool (strict)"("Disabled"=w273) -> ()  [unwired: 2 in, 2 out]
                n582 = property on="SetVoltageB" class="Bool (strict)"("Disabled"=w273) -> ()  [unwired: 2 in, 2 out]
                n583 = property on="SetOutputOffB" class="Bool (strict)"("Disabled"=w273) -> ()  [unwired: 2 in, 2 out]
                n584 = property on="WriteToFile" class="Bool (strict)"("Disabled"=w273) -> ()  [unwired: 2 in, 2 out]
              }
            }
            n585 = local write "Set Output OFF All"(FALSE ("ConnectChannel")) -> ()
          }
        }
      }
      event "WriteToFile": Value Change {
        n586 = event-data() -> ()  [unwired: 7 out]
        n587 = local read "ADRESS"() -> (w275:string[])
        n588 = Array Size(array=w275) -> (size(s)=w274:i32)
        n589 = local read "WriteToFile"() -> (w276:bool)
        n590 = Greater?(x=w274, y=0) -> (0:w278:bool)
        n591 = And(x=w278, y=w276) -> (x .and. y?=w277:bool)
        n592 = flat-sequence {
          tunnel: w277 -> [w281]
          tunnel: w274 -> [w280]
          frame #0 {
            n593 = case shown="True" w281 {
              tunnel: w280 -> [_ w283]
              frame False {
              }
              frame True {
                n594 = Number To Decimal String(number=w283) -> (decimal integer string=w285:string)  [unwired: 1 out]
                n595 = Write to Text File(text=w285) -> (refnum out=w284:refnum<file>, cancelled=w282:bool, error out=w286:errorcluster)  [unwired: 1 in, 2 out]
                n596 = Write to Text File(file (use dialog)=w284, text="\nИМЯ  АДРЕС  НАПРЯЖЕНИЕ  ТОК", error in=w286) -> (refnum out=w287:refnum<file>, error out=w288:errorcluster)  [unwired: 2 out]
                n597 = for {
                  N: w283 -> [_]
                  tunnel: w282 -> [w290]
                  tunnel: w288 -> [w294]
                  tunnel: w287 -> [w292]
                  i -> [w291]
                  w298 = "" ("Control Name")
                  w305 = "\t"
                  n598 = local read "VIRef"() -> (w303:refnum<vi>[])
                  n599 = Index Array(array=w303, index=w291) -> (element=w302:refnum<vi>)
                  n600 = invoke class="VI" method="Ctrl Val.Get"(reference=w302, "Control Name"="SetVoltageStr") -> (reference out=w296:refnum<vi>, "Get Control Value Variant"=w304:variant)  [unwired: 2 in, 2 out]
                  n601 = invoke class="VI" method="Ctrl Val.Get"(reference=w296, "Control Name"="SetCurrentStr") -> ("Get Control Value Variant"=w299:variant)  [unwired: 2 in, 3 out]
                  n602 = local read "ADRESS"() -> (w310:string[])
                  n603 = local read "NAME"() -> (w308:string[])
                  n604 = Variant To Data(type=w298, Variant=w299) -> (data=w295:string)  [unwired: 1 in, 1 out]
                  n605 = Variant To Data(type=w298, Variant=w304) -> (data=w300:string)  [unwired: 1 in, 1 out]
                  n606 = Index Array(array=w308, index=w291) -> (element=w306:string)
                  n607 = Index Array(array=w310, index=w291) -> (element=w309:string)
                  n608 = Concatenate Strings("\r\n", w306, w305, w309, w305, w300, w305, w295) -> (w293:string)
                  n609 = case shown="False" w290 {
                    tunnel: w292 -> [w312 _]
                    tunnel: w293 -> [w313 _]
                    tunnel: w294 -> [w311 _]
                    frame False {
                      n610 = Write to Text File(file (use dialog)=w312, text=w313, error in=w311) -> ()  [unwired: 4 out]
                    }
                    frame True {
                    }
                  }
                }
              }
            }
          }
          frame #1 {
            n611 = local write "WriteToFile"(FALSE ("ConnectChannel")) -> ()
          }
        }
      }
      event "ReadFromFile": Value Change {
        n612 = event-data() -> ()  [unwired: 7 out]
        n613 = Read from Text File(count=100) -> (text=w317:string[], cancelled=w315:bool, error out=w316:errorcluster)  [unwired: 1 in, 3 out]
        n614 = call <vilib>:"Clear Errors.vi"("error in (no error)"=w316) -> ()  [unwired: 7 out]
        n615 = local read "ReadFromFile"() -> (w320:bool)
        n616 = Not(x=w315) -> (.not. x?=w321:bool)
        n617 = And(x=w320, y=w321) -> (x .and. y?=w319:bool)
        n618 = case shown="True" w319 {
          tunnel: w317 -> [_ w344]
          frame False {
            n619 = local write "ReadFromFile"(FALSE ("ConnectChannel")) -> ()
          }
          frame True {
            w323 = T1 0 items=["no dialog", "OK message", "continue or stop message", "OK message + warnings", "continue/stop + warnings"] ("type of dialog (OK msg:1)")
            w343 = u8 2 ("Disabled")
            n620 = flat-sequence {
              tunnel: w344 -> [w362]
              tunnel: [w361] -> w326
              tunnel: w326 -> [w401]
              tunnel: [w401] -> w325
              frame #0 {
                n621 = local read "VIRef"() -> (w345:refnum<vi>[])
                n622 = Array Size(array=w345) -> (size(s)=w346:i32)
                n623 = for {
                  N: w346 -> [_]
                  tunnel: w345 -> [w348]
                  i -> [w349]
                  n624 = Index Array(array=w348, index=w349) -> (element=w347:refnum<vi>)
                  n625 = invoke class="VI" method="Ctrl Val.Set"(reference=w347, "Control Name"="Connect", "Value"=FALSE) -> ()  [unwired: 2 in, 5 out]
                }
              }
              frame #1 {
                n626 = Wait (ms)(milliseconds to wait=u32 2500) -> ()  [unwired: 1 out]
              }
              frame #2 {
                n627 = local read "VIRef"() -> (w354:refnum<vi>[])
                n628 = Array Size(array=w354) -> (size(s)=w353:i32)
                n629 = for {
                  N: w353 -> [_]
                  tunnel: w354 -> [w356]
                  i -> [w357]
                  n630 = Index Array(array=w356, index=w357) -> (element=w355:refnum<vi>)
                  n631 = invoke class="VI" method="Abort VI"(reference=w355) -> ()  [unwired: 2 in, 3 out]
                }
              }
              frame #3 {
                w359 = string[] [] ("GlobalInAdress")
                n632 = Wait (ms)(milliseconds to wait=u32 500) -> ()  [unwired: 1 out]
                n633 = local write "NAME"(w359) -> ()
                n634 = local write "ADRESS"(w359) -> ()
                n635 = local write "VIRef"(refnum<vi>[] []) -> ()
              }
              frame #4 {
                n636 = Index Array(array=w362, index=0) -> (element=w365:string)
                n637 = Decimal String To Number(string=w365) -> (number=w363:i32)  [unwired: 3 out]
                n638 = for {
                  N: w363 -> [_]
                  tunnel: w362 -> [w380]
                  tunnel: [w366] -> w361 mode=indexing
                  i -> [w383]
                  n639 = Add(x=2, y=w383) -> (x+y=w382:i32)
                  n640 = Index Array(array=w380, index=w382) -> (element=w379:string)
                  n641 = Spreadsheet String To Array(format string="%s", spreadsheet string=w379, array type (2D Dbl)=string[] [] ("GlobalInAdress")) -> (array=w370:string[])  [unwired: 1 out]
                  n642 = Index Array(array=w370, index=3) -> (element=w368:string)
                  n643 = Index Array(array=w370, index=0) -> (element=w374:string)
                  n644 = Index Array(array=w370, index=1) -> (element=w375:string)
                  n645 = Index Array(array=w370, index=2) -> (element=w369:string)
                  n646 = flat-sequence {
                    tunnel: w375 -> [w397]
                    tunnel: w374 -> [w398]
                    tunnel: w369 -> [w392]
                    tunnel: w368 -> [w389]
                    tunnel: [w384] -> w367
                    tunnel: [w399] -> w366
                    tunnel: w367 -> [w399]
                    frame #0 {
                      n647 = Scan From String(input string=w389, default 1=0.0 ("default value 1")) -> (output 1=w388:dbl)  [unwired: 3 in, 3 out]
                      n648 = Scan From String(input string=w392, default 1=0.0 ("default value 1")) -> (output 1=w391:dbl)  [unwired: 3 in, 3 out]
                      n649 = local read "ADRESS"() -> (w395:string[])
                      n650 = local read "NAME"() -> (w396:string[])
                      n651 = local read "VIRef"() -> (w394:refnum<vi>[])
                      n652 = call "AddChannel.vi"("VIRef"=w394, "Name"=w398, "SetCurrent"=w388, "ADRESS"=w395, "NAME"=w396, "Address"=w397, "SetVoltage"=w391) -> ("NAMEOut"=w387:string[], "error out"=w384:errorcluster, "ADRESSOut"=w385:string[], "VIRefOut"=w386:refnum<vi>[])  [unwired: 1 in, 4 out]
                      n653 = Build Array (concatenate)(w395, w397) -> ()  [unwired: 1 out]
                      n654 = local write "NAME"(w387) -> ()
                      n655 = local write "ADRESS"(w385) -> ()
                      n656 = local write "VIRef"(w386) -> ()
                    }
                    frame #1 {
                      n657 = Wait (ms)(milliseconds to wait=u32 50) -> ()  [unwired: 1 out]
                    }
                  }
                }
              }
              frame #5 {
                w402 = u8 0 ("Disabled")
                n658 = local write "ReadFromFile"(FALSE ("ConnectChannel")) -> ()
                n659 = property on="Set Output OFF All" class="Bool (strict)"("Disabled"=w402) -> ()  [unwired: 2 in, 2 out]
                n660 = property on="ConnectAll" class="Bool (strict)"("Disabled"=w402) -> ()  [unwired: 2 in, 2 out]
                n661 = property on="Set Output ON All" class="Bool (strict)"("Disabled"=w402) -> ()  [unwired: 2 in, 2 out]
                n662 = property on="AddChannel" class="Bool (strict)"("Disabled"=w402) -> ()  [unwired: 2 in, 2 out]
                n663 = property on="CurrentModulationB" class="Bool (strict)"("Disabled"=w402) -> ()  [unwired: 2 in, 2 out]
                n664 = property on="DisconnectChannel" class="Bool (strict)"("Disabled"=w402) -> ()  [unwired: 2 in, 2 out]
                n665 = property on="ReadFromFile" class="Bool (strict)"("Disabled"=w402) -> ()  [unwired: 2 in, 2 out]
                n666 = property on="ConnectChannel" class="Bool (strict)"("Disabled"=w402) -> ()  [unwired: 2 in, 2 out]
                n667 = property on="DeleteChannel" class="Bool (strict)"("Disabled"=w402) -> ()  [unwired: 2 in, 2 out]
                n668 = property on="WriteToFile" class="Bool (strict)"("Disabled"=w402) -> ()  [unwired: 2 in, 2 out]
                n669 = property on="SetCurrentB" class="Bool (strict)"("Disabled"=w402) -> ()  [unwired: 2 in, 2 out]
                n670 = property on="Quit" class="Bool (strict)"("Disabled"=w402) -> ()  [unwired: 2 in, 2 out]
                n671 = property on="SetOutputOnB" class="Bool (strict)"("Disabled"=w402) -> ()  [unwired: 2 in, 2 out]
                n672 = property on="SetVoltageB" class="Bool (strict)"("Disabled"=w402) -> ()  [unwired: 2 in, 2 out]
                n673 = property on="SetOutputOffB" class="Bool (strict)"("Disabled"=w402) -> ()  [unwired: 2 in, 2 out]
                n674 = property on="SetVoltageAll" class="Bool (strict)"("Disabled"=w402) -> ()  [unwired: 2 in, 2 out]
                n675 = property on="SetCurrentAll" class="Bool (strict)"("Disabled"=w402) -> ()  [unwired: 2 in, 2 out]
                n676 = property on="DisconnectAll" class="Bool (strict)"("Disabled"=w402) -> ()  [unwired: 2 in, 2 out]
              }
            }
            n677 = property on="ConnectAll" class="Bool (strict)"("Disabled"=w343) -> (error out=w342:errorcluster)  [unwired: 2 in, 1 out]
            n678 = property on="DeleteChannel" class="Bool (strict)"("Disabled"=w343) -> (error out=w335:errorcluster)  [unwired: 2 in, 1 out]
            n679 = property on="Set Output OFF All" class="Bool (strict)"(error in=w342, "Disabled"=w343) -> (error out=w341:errorcluster)  [unwired: 1 in, 1 out]
            n680 = property on="WriteToFile" class="Bool (strict)"(error in=w335, "Disabled"=w343) -> (error out=w334:errorcluster)  [unwired: 1 in, 1 out]
            n681 = property on="Set Output ON All" class="Bool (strict)"(error in=w341, "Disabled"=w343) -> (error out=w340:errorcluster)  [unwired: 1 in, 1 out]
            n682 = property on="SetCurrentB" class="Bool (strict)"(error in=w334, "Disabled"=w343) -> (error out=w333:errorcluster)  [unwired: 1 in, 1 out]
            n683 = property on="Quit" class="Bool (strict)"(error in=w333, "Disabled"=w343) -> (error out=w331:errorcluster)  [unwired: 1 in, 1 out]
            n684 = property on="AddChannel" class="Bool (strict)"(error in=w340, "Disabled"=w343) -> (error out=w339:errorcluster)  [unwired: 1 in, 1 out]
            n685 = property on="SetOutputOnB" class="Bool (strict)"(error in=w331, "Disabled"=w343) -> (error out=w332:errorcluster)  [unwired: 1 in, 1 out]
            n686 = property on="CurrentModulationB" class="Bool (strict)"(error in=w339, "Disabled"=w343) -> (error out=w338:errorcluster)  [unwired: 1 in, 1 out]
            n687 = property on="SetVoltageB" class="Bool (strict)"(error in=w332, "Disabled"=w343) -> (error out=w330:errorcluster)  [unwired: 1 in, 1 out]
            n688 = property on="DisconnectChannel" class="Bool (strict)"(error in=w338, "Disabled"=w343) -> (error out=w337:errorcluster)  [unwired: 1 in, 1 out]
            n689 = property on="SetOutputOffB" class="Bool (strict)"(error in=w330, "Disabled"=w343) -> (error out=w328:errorcluster)  [unwired: 1 in, 1 out]
            n690 = property on="ReadFromFile" class="Bool (strict)"(error in=w337, "Disabled"=w343) -> (error out=w336:errorcluster)  [unwired: 1 in, 1 out]
            n691 = property on="SetVoltageAll" class="Bool (strict)"(error in=w328, "Disabled"=w343) -> (error out=w329:errorcluster)  [unwired: 1 in, 1 out]
            n692 = property on="SetCurrentAll" class="Bool (strict)"(error in=w329, "Disabled"=w343) -> (error out=w327:errorcluster)  [unwired: 1 in, 1 out]
            n693 = property on="ConnectChannel" class="Bool (strict)"(error in=w336, "Disabled"=w343) -> ()  [unwired: 1 in, 2 out]
            n694 = property on="DisconnectAll" class="Bool (strict)"(error in=w327, "Disabled"=w343) -> ()  [unwired: 1 in, 2 out]
            n695 = Merge Errors(w325) -> (w324:errorcluster)
            n696 = call <vilib>:"General Error Handler.vi"("type of dialog (OK msg:1)"=w323, "error in (no error)"=w324) -> ()  [unwired: 14 out]
          }
        }
      }
      event "SetCurrentB": Value Change {
        n697 = event-data() -> ()  [unwired: 7 out]
        n698 = property on="List of channels" class="MCListbox (strict)"() -> ("Value"=w404:i32)  [unwired: 2 in, 2 out]
        n699 = local read "SetCurrentB"() -> (w405:bool)
        n700 = Greater Or Equal?(x=w404, y=0) -> (x >= y?=w407:bool)
        n701 = And(x=w407, y=w405) -> (x .and. y?=w406:bool)
        n702 = case shown="True" w406 {
          tunnel: w404 -> [_ w411]
          frame False {
          }
          frame True {
            n703 = flat-sequence {
              tunnel: w411 -> [w413]
              tunnel: [w413] -> w409
              tunnel: w409 -> [w418]
              frame #0 {
                w412 = u8 2 ("Disabled")
                n704 = property on="Quit" class="Bool (strict)"("Disabled"=w412) -> ()  [unwired: 2 in, 2 out]
                n705 = property on="ConnectAll" class="Bool (strict)"("Disabled"=w412) -> ()  [unwired: 2 in, 2 out]
                n706 = property on="Set Output OFF All" class="Bool (strict)"("Disabled"=w412) -> ()  [unwired: 2 in, 2 out]
                n707 = property on="AddChannel" class="Bool (strict)"("Disabled"=w412) -> ()  [unwired: 2 in, 2 out]
                n708 = property on="Set Output ON All" class="Bool (strict)"("Disabled"=w412) -> ()  [unwired: 2 in, 2 out]
                n709 = property on="CurrentModulationB" class="Bool (strict)"("Disabled"=w412) -> ()  [unwired: 2 in, 2 out]
                n710 = property on="DisconnectChannel" class="Bool (strict)"("Disabled"=w412) -> ()  [unwired: 2 in, 2 out]
                n711 = property on="ReadFromFile" class="Bool (strict)"("Disabled"=w412) -> ()  [unwired: 2 in, 2 out]
                n712 = property on="ConnectChannel" class="Bool (strict)"("Disabled"=w412) -> ()  [unwired: 2 in, 2 out]
                n713 = property on="DeleteChannel" class="Bool (strict)"("Disabled"=w412) -> ()  [unwired: 2 in, 2 out]
                n714 = property on="WriteToFile" class="Bool (strict)"("Disabled"=w412) -> ()  [unwired: 2 in, 2 out]
                n715 = property on="SetCurrentB" class="Bool (strict)"("Disabled"=w412) -> ()  [unwired: 2 in, 2 out]
                n716 = property on="SetOutputOnB" class="Bool (strict)"("Disabled"=w412) -> ()  [unwired: 2 in, 2 out]
                n717 = property on="SetVoltageB" class="Bool (strict)"("Disabled"=w412) -> ()  [unwired: 2 in, 2 out]
                n718 = property on="SetOutputOffB" class="Bool (strict)"("Disabled"=w412) -> ()  [unwired: 2 in, 2 out]
                n719 = property on="SetVoltageAll" class="Bool (strict)"("Disabled"=w412) -> ()  [unwired: 2 in, 2 out]
                n720 = property on="SetCurrentAll" class="Bool (strict)"("Disabled"=w412) -> ()  [unwired: 2 in, 2 out]
                n721 = property on="DisconnectAll" class="Bool (strict)"("Disabled"=w412) -> ()  [unwired: 2 in, 2 out]
              }
              frame #1 {
                n722 = local read "VIRef"() -> (w420:refnum<vi>[])
                n723 = local read "SetCurrent"() -> (w417:dbl)
                n724 = Index Array(array=w420, index=w418) -> (element=w419:refnum<vi>)
                n725 = invoke class="VI" method="Ctrl Val.Set"(reference=w419, "Control Name"="SetCurrent", "Value"=w417) -> (reference out=w414:refnum<vi>)  [unwired: 2 in, 4 out]
                n726 = invoke class="VI" method="Ctrl Val.Set"(reference=w414, "Control Name"="NeedToSetCurrent", "Value"=TRUE ("ConnectChannel")) -> ()  [unwired: 2 in, 5 out]
              }
              frame #2 {
                w422 = u8 0 ("Disabled")
                n727 = property on="Quit" class="Bool (strict)"("Disabled"=w422) -> ()  [unwired: 2 in, 2 out]
                n728 = property on="ConnectAll" class="Bool (strict)"("Disabled"=w422) -> ()  [unwired: 2 in, 2 out]
                n729 = property on="Set Output OFF All" class="Bool (strict)"("Disabled"=w422) -> ()  [unwired: 2 in, 2 out]
                n730 = property on="AddChannel" class="Bool (strict)"("Disabled"=w422) -> ()  [unwired: 2 in, 2 out]
                n731 = property on="Set Output ON All" class="Bool (strict)"("Disabled"=w422) -> ()  [unwired: 2 in, 2 out]
                n732 = property on="DisconnectChannel" class="Bool (strict)"("Disabled"=w422) -> ()  [unwired: 2 in, 2 out]
                n733 = property on="ReadFromFile" class="Bool (strict)"("Disabled"=w422) -> ()  [unwired: 2 in, 2 out]
                n734 = property on="ConnectChannel" class="Bool (strict)"("Disabled"=w422) -> ()  [unwired: 2 in, 2 out]
                n735 = property on="DeleteChannel" class="Bool (strict)"("Disabled"=w422) -> ()  [unwired: 2 in, 2 out]
                n736 = property on="DisconnectAll" class="Bool (strict)"("Disabled"=w422) -> ()  [unwired: 2 in, 2 out]
                n737 = property on="CurrentModulationB" class="Bool (strict)"("Disabled"=w422) -> ()  [unwired: 2 in, 2 out]
                n738 = property on="WriteToFile" class="Bool (strict)"("Disabled"=w422) -> ()  [unwired: 2 in, 2 out]
                n739 = property on="SetCurrentB" class="Bool (strict)"("Disabled"=w422) -> ()  [unwired: 2 in, 2 out]
                n740 = property on="SetOutputOnB" class="Bool (strict)"("Disabled"=w422) -> ()  [unwired: 2 in, 2 out]
                n741 = property on="SetVoltageB" class="Bool (strict)"("Disabled"=w422) -> ()  [unwired: 2 in, 2 out]
                n742 = property on="SetOutputOffB" class="Bool (strict)"("Disabled"=w422) -> ()  [unwired: 2 in, 2 out]
                n743 = property on="SetVoltageAll" class="Bool (strict)"("Disabled"=w422) -> ()  [unwired: 2 in, 2 out]
                n744 = property on="SetCurrentAll" class="Bool (strict)"("Disabled"=w422) -> ()  [unwired: 2 in, 2 out]
              }
            }
            n745 = local write "SetCurrentB"(FALSE ("ConnectChannel")) -> ()
          }
        }
      }
      event "CurrentModulationB": Value Change {
        n746 = event-data() -> ()  [unwired: 7 out]
        n747 = local read "CurrentModulationB"() -> (w423:bool)
        n748 = case shown="False" w423 {
          frame False {
            n749 = flat-sequence {
              frame #0 {
                n750 = local write "CurrentModulationOn"(FALSE ("CurrentModulationOn")) -> ()
              }
              frame #1 {
                n751 = Wait (ms)(milliseconds to wait=u32 500) -> ()  [unwired: 1 out]
              }
              frame #2 {
                n752 = local read "VIRef"() -> (w427:refnum<vi>[])
                n753 = Array Size(array=w427) -> (size(s)=w426:i32)
                n754 = for {
                  N: w426 -> [_]
                  i -> [w429]
                  n755 = local read "CURRENTSET"() -> (w430:dbl[])
                  n756 = local read "VIRef"() -> (w435:refnum<vi>[])
                  n757 = Index Array(array=w430, index=w429) -> (element=w428:dbl)
                  n758 = Index Array(array=w435, index=w429) -> (element=w431:refnum<vi>)
                  n759 = invoke class="VI" method="Ctrl Val.Set"(reference=w431, "Control Name"="SetCurrent", "Value"=w428) -> (reference out=w432:refnum<vi>)  [unwired: 2 in, 4 out]
                  n760 = invoke class="VI" method="Ctrl Val.Set"(reference=w432, "Control Name"="NeedToSetCurrent", "Value"=TRUE ("ConnectChannel")) -> ()  [unwired: 2 in, 5 out]
                }
              }
            }
          }
          frame True {
            n761 = flat-sequence {
              frame #0 {
                n762 = local read "VIRef"() -> (w440:refnum<vi>[])
                n763 = local read "Amp"() -> (w443:dbl)
                n764 = local read "Step"() -> (w442:dbl)
                n765 = local write "ModulationState"(0 ("ModulationState")) -> ()
                n766 = local write "ModulationUpDown"(TRUE ("ModulationUpDown")) -> ()
                n767 = Divide(x=w443, y=w442) -> (x/y=w444:dbl)
                n768 = Array Size(array=w440) -> (size(s)=w439:i32)
                n769 = for {
                  N: w439 -> [_]
                  i -> [w448]
                  n770 = local read "VIRef"() -> (w451:refnum<vi>[])
                  n771 = Index Array(array=w451, index=w448) -> (element=w450:refnum<vi>)
                  n772 = invoke class="VI" method="Ctrl Val.Get"(reference=w450, "Control Name"="SetCurrent") -> ("Get Control Value Variant"=w455:variant)  [unwired: 2 in, 3 out]
                  n773 = local read "CURRENTSET"() -> (w449:dbl[])
                  n774 = Variant To Data(type=0.0 ("Amp"), Variant=w455) -> (data=w452:dbl)  [unwired: 1 in, 1 out]
                  n775 = Insert Into Array(array=w449, index=w448, new element=w452) -> (w447:dbl[])
                  n776 = local write "CURRENTSET"(w447) -> ()
                }
                n777 = Round Toward +Infinity(x=w444) -> (ceil(x): smallest int >= x=w441:dbl)
                n778 = Initialize Array(0.0 ("element"), w439) -> (w437:dbl[])
                n779 = local write "CURRENTSET"(w437) -> ()
                n780 = local write "ModulationNumberOfSteps"(w441) -> ()
              }
              frame #1 {
                n781 = local write "CurrentModulationOn"(TRUE ("CurrentModulationOn")) -> ()
              }
            }
          }
        }
      }
      event "DeleteChannel": Value Change {
        w457 = 0 ("y")
        n782 = event-data() -> ()  [unwired: 7 out]
        n783 = property on="List of channels" class="MCListbox (strict)"() -> ("Value"=w461:i32)  [unwired: 2 in, 2 out]
        n784 = local read "DeleteChannel"() -> (w459:bool)
        n785 = Greater Or Equal?(x=w461, y=w457) -> (x >= y?=w460:bool)
        n786 = And(x=w460, y=w459) -> (x .and. y?=w458:bool)
        n787 = case shown="True" w458 {
          tunnel: w457 -> [_ w465]
          frame False {
            n788 = local write "DeleteChannel"(FALSE ("DeleteChannel")) -> ()
          }
          frame True {
            n789 = flat-sequence {
              tunnel: [w474] -> w469
              tunnel: [w473] -> w466
              tunnel: w465 -> [w473]
              tunnel: [w472] -> w464
              tunnel: [w480] -> w470
              tunnel: w469 -> [w480]
              tunnel: [w479] -> w467
              tunnel: w466 -> [w479]
              tunnel: w464 -> [w478]
              tunnel: [w478] -> w463
              tunnel: w470 -> [w485]
              tunnel: [w484] -> w468
              tunnel: w467 -> [w484]
              tunnel: w463 -> [w483]
              tunnel: w468 -> [w486]
              frame #0 {
                w471 = u8 2 ("Disabled")
                n790 = property on="Quit" class="Bool (strict)"("Disabled"=w471) -> ()  [unwired: 2 in, 2 out]
                n791 = property on="ConnectAll" class="Bool (strict)"("Disabled"=w471) -> ()  [unwired: 2 in, 2 out]
                n792 = property on="Set Output OFF All" class="Bool (strict)"("Disabled"=w471) -> ()  [unwired: 2 in, 2 out]
                n793 = property on="AddChannel" class="Bool (strict)"("Disabled"=w471) -> ()  [unwired: 2 in, 2 out]
                n794 = property on="Set Output ON All" class="Bool (strict)"("Disabled"=w471) -> ()  [unwired: 2 in, 2 out]
                n795 = property on="CurrentModulationB" class="Bool (strict)"("Disabled"=w471) -> ()  [unwired: 2 in, 2 out]
                n796 = property on="DisconnectChannel" class="Bool (strict)"("Disabled"=w471) -> ()  [unwired: 2 in, 2 out]
                n797 = property on="ReadFromFile" class="Bool (strict)"("Disabled"=w471) -> ()  [unwired: 2 in, 2 out]
                n798 = property on="ConnectChannel" class="Bool (strict)"("Disabled"=w471) -> ()  [unwired: 2 in, 2 out]
                n799 = property on="DeleteChannel" class="Bool (strict)"("Disabled"=w471) -> ()  [unwired: 2 in, 2 out]
                n800 = property on="WriteToFile" class="Bool (strict)"("Disabled"=w471) -> ()  [unwired: 2 in, 2 out]
                n801 = property on="SetCurrentB" class="Bool (strict)"("Disabled"=w471) -> ()  [unwired: 2 in, 2 out]
                n802 = property on="SetOutputOnB" class="Bool (strict)"("Disabled"=w471) -> ()  [unwired: 2 in, 2 out]
                n803 = property on="SetVoltageB" class="Bool (strict)"("Disabled"=w471) -> ()  [unwired: 2 in, 2 out]
                n804 = property on="SetOutputOffB" class="Bool (strict)"("Disabled"=w471) -> ()  [unwired: 2 in, 2 out]
                n805 = property on="SetVoltageAll" class="Bool (strict)"("Disabled"=w471) -> ()  [unwired: 2 in, 2 out]
                n806 = property on="SetCurrentAll" class="Bool (strict)"("Disabled"=w471) -> ()  [unwired: 2 in, 2 out]
                n807 = property on="DisconnectAll" class="Bool (strict)"("Disabled"=w471) -> ()  [unwired: 2 in, 2 out]
              }
              frame #1 {
                n808 = local read "VIRef"() -> (w476:refnum<vi>[])
                n809 = Index Array(array=w476, index=w473) -> (element=w474:refnum<vi>)
                n810 = invoke class="VI" method="Ctrl Val.Set"(reference=w474, "Control Name"="Connect", "Value"=FALSE ("OK Button")) -> (error out=w472:errorcluster)  [unwired: 2 in, 4 out]
              }
              frame #2 {
                n811 = Wait (ms)(milliseconds to wait=u32 2500) -> ()  [unwired: 1 out]
              }
              frame #3 {
                n812 = invoke class="VI" method="Abort VI"(reference=w485, error in=w483) -> (error out=w482:errorcluster)  [unwired: 1 in, 2 out]
                n813 = call <vilib>:"Clear Errors.vi"("error in (no error)"=w482) -> ()  [unwired: 7 out]
              }
              frame #4 {
                w487 = 1 ("length")
                n814 = local read "NAME"() -> (w488:string[])
                n815 = local read "VIRef"() -> (w493:refnum<vi>[])
                n816 = local read "ADRESS"() -> (w492:string[])
                n817 = Delete From Array(array=w493, length=w487, index=w486) -> (array with subset deleted=w490:refnum<vi>[])  [unwired: 1 out]
                n818 = Delete From Array(array=w488, length=w487, index=w486) -> (array with subset deleted=w489:string[])  [unwired: 1 out]
                n819 = local write "NAME"(w489) -> ()
                n820 = local write "VIRef"(w490) -> ()
                n821 = Delete From Array(array=w492, length=w487, index=w486) -> (array with subset deleted=w491:string[])  [unwired: 1 out]
                n822 = local write "ADRESS"(w491) -> ()
              }
              frame #5 {
                w494 = u8 0 ("Disabled")
                n823 = local write "DeleteChannel"(FALSE ("DeleteChannel")) -> ()
                n824 = property on="Quit" class="Bool (strict)"("Disabled"=w494) -> ()  [unwired: 2 in, 2 out]
                n825 = property on="Set Output OFF All" class="Bool (strict)"("Disabled"=w494) -> ()  [unwired: 2 in, 2 out]
                n826 = property on="ConnectAll" class="Bool (strict)"("Disabled"=w494) -> ()  [unwired: 2 in, 2 out]
                n827 = property on="AddChannel" class="Bool (strict)"("Disabled"=w494) -> ()  [unwired: 2 in, 2 out]
                n828 = property on="CurrentModulationB" class="Bool (strict)"("Disabled"=w494) -> ()  [unwired: 2 in, 2 out]
                n829 = property on="DisconnectChannel" class="Bool (strict)"("Disabled"=w494) -> ()  [unwired: 2 in, 2 out]
                n830 = property on="ReadFromFile" class="Bool (strict)"("Disabled"=w494) -> ()  [unwired: 2 in, 2 out]
                n831 = property on="ConnectChannel" class="Bool (strict)"("Disabled"=w494) -> ()  [unwired: 2 in, 2 out]
                n832 = property on="DeleteChannel" class="Bool (strict)"("Disabled"=w494) -> ()  [unwired: 2 in, 2 out]
                n833 = property on="SetOutputOffB" class="Bool (strict)"("Disabled"=w494) -> ()  [unwired: 2 in, 2 out]
                n834 = property on="Set Output ON All" class="Bool (strict)"("Disabled"=w494) -> ()  [unwired: 2 in, 2 out]
                n835 = property on="SetVoltageAll" class="Bool (strict)"("Disabled"=w494) -> ()  [unwired: 2 in, 2 out]
                n836 = property on="SetCurrentAll" class="Bool (strict)"("Disabled"=w494) -> ()  [unwired: 2 in, 2 out]
                n837 = property on="DisconnectAll" class="Bool (strict)"("Disabled"=w494) -> ()  [unwired: 2 in, 2 out]
                n838 = property on="WriteToFile" class="Bool (strict)"("Disabled"=w494) -> ()  [unwired: 2 in, 2 out]
                n839 = property on="SetCurrentB" class="Bool (strict)"("Disabled"=w494) -> ()  [unwired: 2 in, 2 out]
                n840 = property on="SetOutputOnB" class="Bool (strict)"("Disabled"=w494) -> ()  [unwired: 2 in, 2 out]
                n841 = property on="SetVoltageB" class="Bool (strict)"("Disabled"=w494) -> ()  [unwired: 2 in, 2 out]
              }
            }
          }
        }
      }
    }
    n842 = Wait (ms)(milliseconds to wait=u32 100) -> ()  [unwired: 1 out]
  }
  n843 = event shown="[0] \"Quit\": Value Change" {
    selector: _ -> [_]
    dyn-events: _ -> [_]
    timeout: _ -> [_]
    event "Quit": Value Change {
      n844 = event-data() -> ()  [unwired: 7 out]
      n845 = local read "Quit"() -> (w496:bool)
      n846 = case shown="True" w496 {
        frame False {
        }
        frame True {
          n847 = flat-sequence {
            frame #0 {
              n848 = local read "VIRef"() -> (w497:refnum<vi>[])
              n849 = Array Size(array=w497) -> (size(s)=w498:i32)
              n850 = for {
                N: w498 -> [_]
                tunnel: w497 -> [w500]
                i -> [w501]
                n851 = Index Array(array=w500, index=w501) -> (element=w499:refnum<vi>)
                n852 = invoke class="VI" method="Ctrl Val.Set"(reference=w499, "Control Name"="Connect", "Value"=FALSE) -> ()  [unwired: 2 in, 5 out]
              }
            }
            frame #1 {
              n853 = Wait (ms)(milliseconds to wait=u32 2500) -> ()  [unwired: 1 out]
            }
            frame #2 {
              n854 = local read "VIRef"() -> (w506:refnum<vi>[])
              n855 = Array Size(array=w506) -> (size(s)=w505:i32)
              n856 = for {
                N: w505 -> [_]
                tunnel: w506 -> [w508]
                i -> [w509]
                n857 = Index Array(array=w508, index=w509) -> (element=w507:refnum<vi>)
                n858 = invoke class="VI" method="Abort VI"(reference=w507) -> ()  [unwired: 2 in, 3 out]
              }
            }
            frame #3 {
              n859 = Wait (ms)(milliseconds to wait=u32 500) -> ()  [unwired: 1 out]
            }
            frame #4 {
              n860 = local write "Quit"(FALSE ("Quit")) -> ()
              n861 = Stop(stop? (T)=TRUE) -> ()
            }
          }
        }
      }
    }
  }
  n862 = while {
    stop <- FALSE stop-if-true
    n863 = property on="List of channels" class="MCListbox (strict)" props=["Value"]() -> ()  [unwired: 2 in, 3 out]
    n864 = property on="AddChannel" class="Bool (strict)"() -> ("Disabled"=w520:u8)  [unwired: 2 in, 2 out]
    n865 = Wait Until Next ms Multiple(millisecond multiple=u32 250) -> ()  [unwired: 1 out]
    n866 = local read "Quit"() -> (w518:bool)
    n867 = Not(x=w518) -> (.not. x?=w517:bool)
    n868 = Equal?(x=w520, y=u8 0) -> (x = y?=w516:bool)
    n869 = And(x=w517, y=w516) -> (x .and. y?=w515:bool)
    n870 = case shown="True" w515 {
      frame False {
      }
      frame True {
        w523 = string[] [] ("GlobalInAdress")
        n871 = local read "VIRef"() -> (w534:refnum<vi>[])
        n872 = Array Size(array=w534) -> (size(s)=w521:i32)
        n873 = for {
          N: w521 -> [_]
          tunnel: w534 -> [w587]
          shift-right: [w585] -> w531
          shift-left: w523 -> [w584]
          shift-right: [w582] -> w530
          shift-left: w523 -> [w583]
          shift-right: [w573] -> w529
          shift-left: w523 -> [w574]
          shift-right: [w559] -> w528
          shift-left: w523 -> [w569]
          shift-right: [w565] -> w526
          shift-left: w523 -> [w536]
          shift-right: [w557] -> w525
          shift-left: w523 -> [w558]
          shift-right: [w551] -> w522
          shift-left: w523 -> [w554]
          i -> [w586]
          w553 = FALSE
          w556 = "" ("Control Name")
          n874 = Index Array(array=w587, index=w586) -> (element=w535:refnum<vi>)
          n875 = disable-structure shown="Disabled" {
            disable-tunnel: w535 -> [w591 _]
            frame Disabled {
              w589 = "m1" ("Control Name")
              n876 = invoke class="VI" method="Ctrl Val.Get"(reference=w591, "Control Name"=w589) -> ("Get Control Value Variant"=w590:variant)  [unwired: 2 in, 3 out]
              n877 = Variant To Data(type=w589, Variant=w590) -> (data=w588:string)  [unwired: 1 in, 1 out]
            }
            frame Enabled {
            }
          }
          n878 = invoke class="VI" method="Ctrl Val.Get"(reference=w535, "Control Name"="Error") -> (error out=w541:errorcluster, "Get Control Value Variant"=w537:variant)  [unwired: 2 in, 2 out]
          n879 = invoke class="VI" method="Ctrl Val.Get"(reference=w535, "Control Name"="GetCurrent") -> (error out=w549:errorcluster, "Get Control Value Variant"=w579:variant)  [unwired: 2 in, 2 out]
          n880 = invoke class="VI" method="Ctrl Val.Get"(reference=w535, "Control Name"="GetVoltage") -> (error out=w548:errorcluster, "Get Control Value Variant"=w580:variant)  [unwired: 2 in, 2 out]
          n881 = invoke class="VI" method="Ctrl Val.Get"(reference=w535, "Control Name"="SetVoltageStr") -> (error out=w547:errorcluster, "Get Control Value Variant"=w572:variant)  [unwired: 2 in, 2 out]
          n882 = invoke class="VI" method="Ctrl Val.Get"(reference=w535, "Control Name"="SetCurrentStr") -> (error out=w546:errorcluster, "Get Control Value Variant"=w571:variant)  [unwired: 2 in, 2 out]
          n883 = invoke class="VI" method="Ctrl Val.Get"(reference=w535, "Control Name"="Output") -> (error out=w545:errorcluster, "Get Control Value Variant"=w560:variant)  [unwired: 2 in, 2 out]
          n884 = invoke class="VI" method="Ctrl Val.Get"(reference=w535, "Control Name"="Active") -> (error out=w544:errorcluster, "Get Control Value Variant"=w568:variant)  [unwired: 2 in, 2 out]
          n885 = Variant To Data(type=w553, Variant=w568) -> (data=w566:bool)  [unwired: 1 in, 1 out]
          n886 = Variant To Data(type=w553, Variant=w537) -> (data=w552:bool)  [unwired: 1 in, 1 out]
          n887 = Merge Errors(w549, w548, w547) -> (w543:errorcluster)
          n888 = Merge Errors(w546, w545, w544) -> (w542:errorcluster)
          n889 = Variant To Data(type=w556, Variant=w579) -> (data=w576:string)  [unwired: 1 in, 1 out]
          n890 = Variant To Data(type=w556, Variant=w580) -> (data=w577:string)  [unwired: 1 in, 1 out]
          n891 = Variant To Data(type=w556, Variant=w572) -> (data=w563:string)  [unwired: 1 in, 1 out]
          n892 = Variant To Data(type=w556, Variant=w571) -> (data=w562:string)  [unwired: 1 in, 1 out]
          n893 = Variant To Data(type=w556, Variant=w560) -> (data=w539:string)  [unwired: 1 in, 1 out]
          n894 = Merge Errors(w543, w542, w541) -> (w540:errorcluster)
          n895 = Build Array (concatenate)(w583, w576) -> (w582:string[])
          n896 = Build Array (concatenate)(w584, w577) -> (w585:string[])
          n897 = Build Array (concatenate)(w574, w563) -> (w573:string[])
          n898 = Build Array (concatenate)(w569, w562) -> (w559:string[])
          n899 = case shown="True" w552 {
            tunnel: ["" ("Control Name") "ERROR" ("Control Name")] -> w550
            tunnel: w535 -> [_ w594]
            frame False {
            }
            frame True {
              n900 = case shown="True" "Boolean" {
                tunnel: w594 -> [_ w605]
                frame False {
                }
                frame True {
                  w598 = T1 0 items=["no dialog", "OK message", "continue or stop message", "OK message + warnings", "continue/stop + warnings"] ("type of dialog (OK msg:1)")
                  w597 = "Connect" ("Control Name")
                  n901 = invoke class="VI" method="Ctrl Val.Set"(reference=w605, "Control Name"=w597, "Value"=FALSE ("OK Button")) -> (reference out=w601:refnum<vi>, error out=w604:errorcluster)  [unwired: 2 in, 3 out]
                  n902 = flat-sequence {
                    tunnel: w604 -> [w610]
                    tunnel: [w610] -> w602
                    tunnel: w601 -> [w608]
                    tunnel: [w608] -> w600
                    tunnel: w597 -> [w607]
                    tunnel: [w607] -> w596
                    frame #0 {
                      n903 = Wait (ms)(milliseconds to wait=u32 1000) -> ()  [unwired: 1 out]
                    }
                  }
                  n904 = invoke class="VI" method="Ctrl Val.Set"(reference=w600, error in=w602, "Control Name"=w596, "Value"=TRUE ("OK Button")) -> (error out=w599:errorcluster)  [unwired: 1 in, 4 out]
                  n905 = call <vilib>:"General Error Handler.vi"("type of dialog (OK msg:1)"=w598, "error in (no error)"=w599) -> ()  [unwired: 14 out]
                }
              }
            }
          }
          n906 = case shown="\"1\"" w539 {
            tunnel: ["ON" ("Control Name") "" ("Control Name") "OFF" ("Control Name")] -> w538
            frame "1" {
            }
            frame Default {
            }
            frame "0" {
            }
          }
          n907 = case shown="True" w566 {
            tunnel: ["No" ("Control Name") "Yes" ("Control Name")] -> w567
            frame False {
            }
            frame True {
            }
          }
          n908 = call <vilib>:"Clear Errors.vi"("error in (no error)"=w540) -> ()  [unwired: 7 out]
          n909 = Build Array (concatenate)(w558, w538) -> (w557:string[])
          n910 = Build Array (concatenate)(w536, w567) -> (w565:string[])
          n911 = Build Array (concatenate)(w554, w550) -> (w551:string[])
        }
        n912 = local read "ADRESS"() -> (w532:string[])
        n913 = local read "NAME"() -> (w527:string[])
        n914 = Build Array(w527, w532, w531, w530, w529, w528, w525, w526, w522) -> (w533:string[][])
        n915 = Transpose 2D Array(2D array=w533) -> (transposed array=w524:string[][])
        n916 = property on="List of channels" class="MCListbox (strict)"("ItemNames"=w524) -> ()  [unwired: 2 in, 2 out]
      }
    }
  }
  n917 = while {
    stop <- FALSE stop-if-true
    n918 = local read "CurrentModulationOn"() -> (w618:bool)
    n919 = Wait Until Next ms Multiple(millisecond multiple="Period") -> ()  [unwired: 1 out]
    n920 = property on="List of channels" class="MCListbox (strict)"() -> ("Value"=w619:i32)  [unwired: 2 in, 2 out]
    n921 = Greater Or Equal?(x=w619, y=0) -> (x >= y?=w617:bool)
    n922 = And(x=w618, y=w617) -> (x .and. y?=w616:bool)
    n923 = case shown="True" w616 {
      frame False {
      }
      frame True {
        n924 = flat-sequence {
          frame #0 {
            n925 = case shown="False" "ModulationUpDown" {
              frame False {
                n926 = local read "ModulationNumberOfSteps"() -> (w625:i32)
                n927 = local read "ModulationState"() -> (w628:i32)
                n928 = Subtract(x=0, y=w625) -> (x-y=w624:i32)
                n929 = Greater?(x=w628, y=w624) -> (0:w627:bool)
                n930 = case shown="False" w627 {
                  frame False {
                    n931 = local read "ModulationState"() -> (w630:i32)
                    n932 = local write "ModulationUpDown"(TRUE ("ModulationUpDown")) -> ()
                    n933 = Increment(x=w630) -> (x+1=w631:i32)
                    n934 = local write "ModulationState"(w631) -> ()
                  }
                  frame True {
                    n935 = local read "ModulationState"() -> (w633:i32)
                    n936 = Decrement(x=w633) -> (x-1=w632:i32)
                    n937 = local write "ModulationState"(w632) -> ()
                  }
                }
              }
              frame True {
                n938 = local read "ModulationNumberOfSteps"() -> (w635:i32)
                n939 = local read "ModulationState"() -> (w636:i32)
                n940 = Less?(x=w636, y=w635) -> (x < y?=w634:bool)
                n941 = case shown="False" w634 {
                  frame False {
                    n942 = local read "ModulationState"() -> (w638:i32)
                    n943 = local write "ModulationUpDown"(FALSE ("ModulationUpDown")) -> ()
                    n944 = Decrement(x=w638) -> (x-1=w639:i32)
                    n945 = local write "ModulationState"(w639) -> ()
                  }
                  frame True {
                    n946 = local read "ModulationState"() -> (w641:i32)
                    n947 = Increment(x=w641) -> (x+1=w640:i32)
                    n948 = local write "ModulationState"(w640) -> ()
                  }
                }
              }
            }
          }
          frame #1 {
            n949 = local read "ModulationState"() -> (w646:i32)
            n950 = local read "CURRENTSET"() -> (w644:dbl[])
            n951 = property on="List of channels" class="MCListbox (strict)"() -> ("Value"=w642:i32)  [unwired: 2 in, 2 out]
            n952 = local read "VIRef"() -> (w653:refnum<vi>[])
            n953 = Multiply(x="Step", y=w646) -> (x*y=w648:dbl)
            n954 = Index Array(array=w644, index=w642) -> (element=w643:dbl)
            n955 = Add(x=w643, y=w648) -> (x+y=w645:dbl)
            n956 = Index Array(array=w653, index=w642) -> (element=w649:refnum<vi>)
            n957 = invoke class="VI" method="Ctrl Val.Set"(reference=w649, "Control Name"="SetCurrent", "Value"=w645) -> (reference out=w650:refnum<vi>)  [unwired: 2 in, 4 out]
            n958 = invoke class="VI" method="Ctrl Val.Set"(reference=w650, "Control Name"="NeedToSetCurrent", "Value"=TRUE ("ConnectChannel")) -> ()  [unwired: 2 in, 5 out]
          }
        }
      }
    }
  }
  n959 = flat-sequence {
    frame #0 {
      n960 = property on="List of channels" class="MCListbox (strict)"("NumRows"=u32 100 ("Number of Rows")) -> ()  [unwired: 2 in, 2 out]
    }
    frame #1 {
      n961 = property on="List of channels" class="MCListbox (strict)"("Height"=u32 465 ("Size:Height")) -> ()  [unwired: 2 in, 2 out]
    }
  }
  n962 = property on="Set Output ON All" class="Bool (strict)"("Disabled"=w17) -> (error out=w7:errorcluster)  [unwired: 2 in, 1 out]
  n963 = property on="AddChannel" class="Bool (strict)"("Disabled"=w17) -> (error out=w16:errorcluster)  [unwired: 2 in, 1 out]
  n964 = property on="AddChannel" class="Bool (strict)"("Disabled"=u8 0) -> ()  [unwired: 2 in, 2 out]
  n965 = local write "WriteToFile"(w20) -> ()
  n966 = local write "DisconnectChannel"(w20) -> ()
  n967 = local write "ConnectChannel"(w20) -> ()
  n968 = local write "SetCurrentB"(w20) -> ()
  n969 = local write "ReadFromFile"(w20) -> ()
  n970 = local write "AddChannel"(w20) -> ()
  n971 = local write "Quit"(w20) -> ()
  n972 = local write "SetCurrentAll"(w20) -> ()
  n973 = local write "SetVoltageAll"(w20) -> ()
  n974 = local write "DeleteChannel"(w20) -> ()
  n975 = local write "SetVoltageB"(w20) -> ()
  n976 = local write "SetOutputOnB"(w19) -> ()
  n977 = local write "ConnectAll"(w19) -> ()
  n978 = local write "SetOutputOffB"(w19) -> ()
  n979 = local write "DisconnectAll"(w19) -> ()
  n980 = local write "CurrentModulationB"(w19) -> ()
  n981 = local write "CurrentModulationOn"(w19) -> ()
  n982 = property on="CurrentModulationB" class="Bool (strict)"(error in=w16, "Disabled"=w17) -> (error out=w15:errorcluster)  [unwired: 1 in, 1 out]
  n983 = property on="DisconnectAll" class="Bool (strict)"(error in=w7, "Disabled"=w17) -> (error out=w6:errorcluster)  [unwired: 1 in, 1 out]
  n984 = property on="DisconnectChannel" class="Bool (strict)"(error in=w15, "Disabled"=w17) -> (error out=w14:errorcluster)  [unwired: 1 in, 1 out]
  n985 = property on="WriteToFile" class="Bool (strict)"(error in=w6, "Disabled"=w17) -> (error out=w5:errorcluster)  [unwired: 1 in, 1 out]
  n986 = property on="SetCurrentB" class="Bool (strict)"(error in=w5, "Disabled"=w17) -> (error out=w4:errorcluster)  [unwired: 1 in, 1 out]
  n987 = property on="ConnectAll" class="Bool (strict)"(error in=w14, "Disabled"=w17) -> (error out=w13:errorcluster)  [unwired: 1 in, 1 out]
  n988 = property on="Quit" class="Bool (strict)"(error in=w4, "Disabled"=w17) -> (error out=w3:errorcluster)  [unwired: 1 in, 1 out]
  n989 = property on="ReadFromFile" class="Bool (strict)"(error in=w13, "Disabled"=w17) -> (error out=w12:errorcluster)  [unwired: 1 in, 1 out]
  n990 = property on="SetOutputOnB" class="Bool (strict)"(error in=w3, "Disabled"=w17) -> (error out=w2:errorcluster)  [unwired: 1 in, 1 out]
  n991 = property on="ConnectChannel" class="Bool (strict)"(error in=w12, "Disabled"=w17) -> (error out=w11:errorcluster)  [unwired: 1 in, 1 out]
  n992 = property on="SetVoltageB" class="Bool (strict)"(error in=w2, "Disabled"=w17) -> (error out=w1:errorcluster)  [unwired: 1 in, 1 out]
  n993 = property on="SetOutputOffB" class="Bool (strict)"(error in=w1, "Disabled"=w17) -> ()  [unwired: 1 in, 2 out]
  n994 = property on="DeleteChannel" class="Bool (strict)"(error in=w11, "Disabled"=w17) -> (error out=w10:errorcluster)  [unwired: 1 in, 1 out]
  n995 = property on="SetVoltageAll" class="Bool (strict)"(error in=w10, "Disabled"=w17) -> (error out=w9:errorcluster)  [unwired: 1 in, 1 out]
  n996 = property on="Set Output OFF All" class="Bool (strict)"(error in=w9, "Disabled"=w17) -> (error out=w8:errorcluster)  [unwired: 1 in, 1 out]
  n997 = property on="SetCurrentAll" class="Bool (strict)"(error in=w8, "Disabled"=w17) -> ()  [unwired: 1 in, 2 out]
  "VIRef" <- refnum<vi>[] []
  "ADRESS" <- string[] [] ("GlobalInAdress")
  "NAME" <- string[] [] ("GlobalInAdress")
  "CURRENTSET" <- dbl[] [] ("GlobalInAdress")
